vi "Forebrain - Final.vi"() -> ()   [LabVIEW 2012]
doc: "This VI contrains the Forebrain within the Olin Robot Architecture. It must be run first to load the appropriate mission definition files. It contains a finite state machine built around a tabbed Operator interface that will guide an operator through the startup, run shutdown mission sequence. After running it, run the Midbrain and Hindbrain VIS."
panel:
  in  "Batshit Velocity":i16
  in  "Alt Rudder":dbl=10.0
  in  "Default Rudder":dbl=9.0
  in  "Max Radius":dbl=300.0
  in  "Battshit":bool
  out "Battery Level":dbl
  in  "MapDarWithBuoys?":bool
  out "under cloud?":bool
  out "WhatAroundMeMap? Filtered":cluster{"T":dbl, "Range":dbl, "Bearing":dbl}[](array[cluster])
  out "Forebrain to Midbrain":T1
  in  "Upper Midbrain Active":bool=TRUE
  out "Ir distance":i16
  in  "Midbrain Behavior weights":i8[](array[numeric])=[10, 0, 0, 0, 0, 0]
  in  "SOFT E-STOP":bool
  in  "Upper Midbrain Tweaks":T2={"Lider good scale mult"=0.00125, "Lider good scale add"=0.0, "Lider speed scale mult"=0.018, "Lider speed scale add"=0.0, "Follow right?"=FALSE, "IR Following Distance"=400, "IR scaling div"=50.0, "Lidar Cutoff"=0.0}
  out "Normalized Buoy Array":i32[][](array[numeric])
  in  "Buoy Array":i32[][](array[numeric])
  out "Number Waypoints":i32
  out "NXT String Sent":string="$B^"
  in  "Soft E-Stop":bool
  out "NXT String Received":string
  out "return count":u32
  out "error out":errorcluster
  in  "error in 2":errorcluster
  out "Desired \nVelocity":i16=5
  out "Ycurrent":dbl format="%#_3g"
  out "Xcurrent":dbl format="%#_3g"
  out "Ystart":dbl
  out "Xstart":dbl
  in  "error in":errorcluster
  out "Robot Live":bool
  in  "E-Stop":bool
  in  "Tab":T3(tab)
  out "MissionTime (Min)":dbl(knob) scale=0.0..10.0
  out "LidarDist":i16
  out "IR Index":i32
  out "BatteryLevel":dbl(slide) scale=6.0..9.0
  out "String Received":string
  out "Send String":string="$B^"
  in  "VISA resource name":refnum<visa-resource-name>="COM6"
  in  "Mode":i16 min=0 max=99 step=1
  in  "Desired Vel":i16(slide)=7 scale=0.0..14.0
  in  "Local Head":i16(slide)=7 scale=0.0..14.0
  out "StartMissionMap":picture
  out "MapDARCheck":picture
  in  "RunRobot":bool
  in  "Tug letter":string="T"
  out "Tug X":i32
  out "Tug Y":i32
  out "Tug H":i32
  out "BS Time Out?":bool
  out "Buoy locations":cluster{"regular expression":string, i32, i32}[](array[cluster])
  out "Valid ?":bool
  out "Battery\nVolts":i16
  out "Base Station data rec'd":string
  out "udp rate":bool
  out "CollisionWarning":bool
  out "DebugMapDAR":picture
  in  "MapDAR Control":T4={"NumberOfBeams"=180, "SensorRange"=500.0, "Noise (0.1 to 1)"=0.0} {"Noise (0.1 to 1)" min=0.0 max=1.0 step=0.1; "SensorRange" min=500.0 max=1500.0 step=100.0; "NumberOfBeams" min=36 max=360 step=2}
  out "MapDAR Data (r:pixel b:degrees)":cluster{"Range":dbl, "Bearing":dbl}[](array[cluster])
  in  "Stop DebugSENSE":bool
  out "MissionMap":picture
  out "Tug position":T5
  out "initialized MDF":T6(array[cluster])
  out "Way Point Index":i32
  out "InitialWaypoint":cluster{"X":i16, "Y":i16}
  in  "Pen Color":u32(colorbox)=15671808
  in  "Select Pen Attributes":T7={"Width"=1, "Style"=enum."Solid"}
  out "Draw??":bool
  in  "WhereAmI?FromBase":T8
  out "(xr,yr)":cluster{"X":dbl, "Y":dbl}
  in  "RobotPosition":T5 {"xrobot" min=0.0 max=1177.0 step=10.0; "yrobot" min=0.0 max=850.0 step=10.0; "heading" min=0.0 max=7.0 step=0.1}
  out "MDF_Original":T6(array[cluster])
  out "WhatAroundMeMap?":cluster{"T":dbl, "Range":dbl, "Bearing":dbl}[](array[cluster])
  out "WayPointAct":dbl[](array[numeric])
  out "SteerAngle":dbl
  out "MissionDefFile":picture
  out "MDF":T6(array[cluster])
  in  "Select Your Behavior":T9(ring)
  out "No. of Waypoints":i32
  in  "Exit Planning":bool
  in  "BoatSpeed for Leg":dbl(slide)=8.0 min=-9.0 max=9.0 step=1.0 scale=0.0..14.0
  out "BuildMDF":bool
  out "WayPoint Position":cluster{"X":i32, "Y":i32}
  out "Send String to NXT":string="$B^"
  in  "Behavior Command":T9(ring)
  out "CollisionLight":bool
  out "Where? Manual":T8
  out "ActManual":bool
  in  "Manual Heading":i16(knob)=7 min=0 max=14 step=1
  out "MWhat?":bool
  out "Where? 2":bool
  out "How? 2":bool
  in  "ManualModeStop":bool
  out "ManualModeMapDAR":picture
  out "ManualMissionMap":picture
  out "Battery":dbl(slide) scale=0.0..8.0
  in  "Manual Vel":dbl(slide)=7.0 min=0.0 max=14.0 step=1.0 scale=0.0..14.0
  out "MissionTime":dbl(knob) scale=0.0..10.0
  out "Heading":cluster{dbl, dbl}(knob)={0.0, 34.390870865624734} scale=180.0..-179.0 scale format="%#_3g"
  out "Speed":i16(knob) scale=-6.0..6.0
  out "Current Behavior":T9(ring)
  out "Robot Position":cluster{"X":dbl, "Y":dbl} {"X" format="%#_3g"; "Y" format="%#_3g"}
  out "Ready":bool
  in  "Pause":bool
  in  "Rerun MDF":bool
  out "CollisionLight 2":bool
  out "Act":bool
  out "Neo-C":bool
  out "How?":bool
  out "What?":bool
  out "A Heading":cluster{dbl, dbl}(knob)={0.0, 34.390870865624734} scale=180.0..-180.0
  out "A Speed":dbl(knob) scale=-9.0..9.0
  out "AutoBattery":dbl(slide) scale=0.0..8.0
  out "AutoModeLIDAR":picture
  out "AutoMissionMap":picture
  in  "RunAutoMode":bool
  out "MissionTimeAuto":dbl(knob) scale=0.0..60.0
  out "Where?":bool
  in  "MISSION NUMBER (1 OR 2)":dbl=1.0
  in  "Mission 2":i64[][](array[numeric])=[[0, 525, 450, 525], [50, 275, 250, 275], [240, 250, 650, 250], [500, 605, 900, 650], [550, 940, 700, 940]]
  in  "WAYPOINT MODE":dbl=1.0
  in  "Current Waypoint":dbl
  in  "Manual\nOverride":bool=TRUE
  in  "Mission 1":i64[][](array[numeric])=[[120, 280, 700, 408], [30, 280, 250, 400], [100, 575, 450, 575], [175, 950, 600, 950]]
  out "BAM Mission Map":picture
  out "Pixel X":dbl
  out "Pixel Y":dbl
  out "Direction":dbl
  out "Base Station String":string
  in  "Heading":i16(knob)=7
  in  "Velocity":i16(slide)=7 scale=0.0..14.0
  out "Local\nHeading":i16=90
  # "To run\nrobot,\nclick\narrow\nabove\n\nRun Robot button must be on"
  # "Operation Directions\n\n1)Click on Startup&\nShutdown tab.\n2) Click on Run \nArrow on menubar.\nRun Forebrain,\nvis from the project\nexplorer.\n3) Select a mssion \nmap file when asked.\n4) Check robot is \nfully operational on\nStartup tab.\n5) Debug with debug\ntabs as required.\n6) Select ManualMode\ntab and test drive \nrobot.\n7) Select PlanMission\ntab and set up \nmission.\n8) Go to AutoMode\ntab and run mission."
  # "BATSHIT PROTOCOL"
  # "Turns off drive\nmotors"
  # "forebrain"
  # "wall follow"
  # "wall avoid"
  # "under cloud"
  # "GTFO"
  # "tend straight"
  # "IR wall avoid"
  # "inactive behaviors = 0\nstrongest behavior = 10"
  # "under cloud should always be zero"
  # "under cloud?"
  # "Enter Olin Test  Pool"
  # "Xbee Com Port"
  # "xBee\"Send String\" (mode, desired velocity, local heading)"
  # "(Type in Tug Letter  L T G P  (look at boat cradle)"
  # "Should be on to\nrun"
  # "BoatG,X,Y,H,BoatT,X,Y,H,BoatP,X,Y.H,BoatL,X,Y,H,BuoyA,X,Y,BuoyB,X,Y,BuoyC,X,Y,BuoyD,X,Y,Time(hours,Min,Sec)"
  # "To stop  program \nturn off here"
  # "Use this tab\nto explore\nLIDAR\ndata and \noperation"
  # "Set\nNumberOfBeams\nSensorRange\nNoise\nto\nview\nsimulated\nsensor\ndata"
  # "Turn Debug Sim \nto leave this\ntab--->"
  # "This tab will auto\nreturn to Startup \nin 2 seconds"
  # "Clean up interface and make more useful for debugging behaviors"
  # "Build out interface and make more useful for debugging act"
  # "This tab will auto\nreturn to Startup \nin 2 seconds"
  # "Directions:\n1) Select Robot Behavior for each mission leg.\n2) Select Robot Speed for leg.\n3) Click on robots current location for first waypoint.\n4) Hold down button and drag to next\nwaypoint. Click on next leg waypoint.\n5) Hold mouse button down and drag to \nnext waypoint. \n6) Click on next waypoint. Repeat for full mission.\n7) MDF will store up to 20 waypoints."
  # "Remember to\nset boat\nleg speed !"
  # "Please Adjust Scroll Barrs in Tug Off Mode to Prevent  Extra Lines Being Drawn"
  # "\"Send String\" (mode, desired velocity, local heading)"
  # "Press to stop and return to StartUp"
  # "Open MidBrain\nArbiter to see\nBrain Waves"
  # "AutoMode\nAutomatically \nReturns to \nStartUp Mode"
  # "LOCATION"
  # "MANUAL CONTROL"
  # "Pixel coordinates for destinations."
  # "BoatG,X,Y,H,BoatT,X,Y,H,BoatP,X,Y.H,BoatL,X,Y,H,BuoyA,X,Y,BuoyB,X,Y,BuoyC,X,Y,BuoyD,X,Y,Time(hours,Min,Sec)"
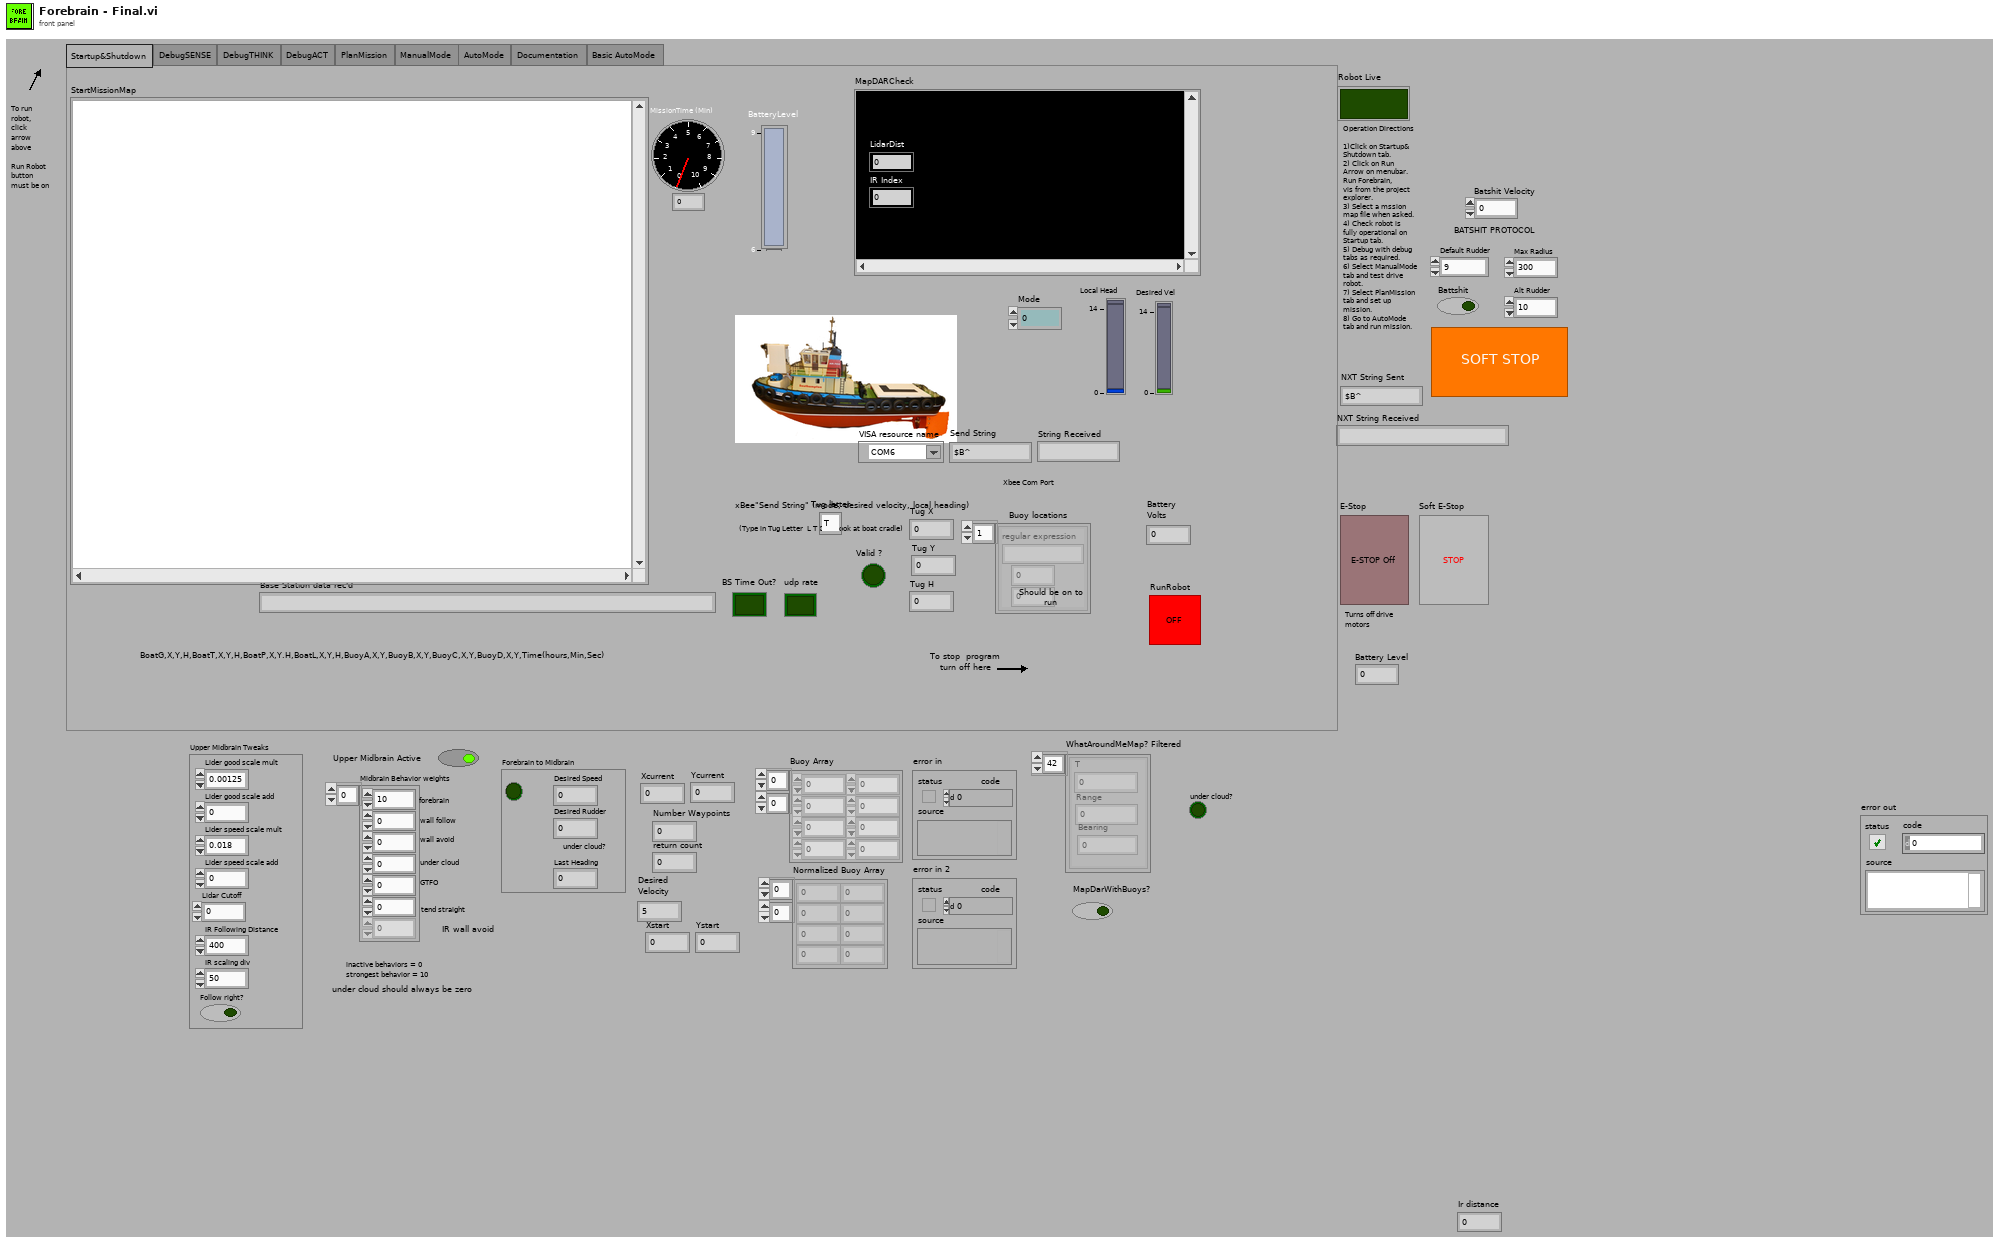
[diagram p1: front panel]
types:
  T1 = cluster{"Desired Speed":i16, "Desired Rudder":i16, bool, "Last Heading":i16}
  T2 = cluster{"Lider good scale mult":dbl, "Lider good scale add":dbl, "Lider speed scale mult":dbl, "Lider speed scale add":dbl, "Follow right?":bool, "IR Following Distance":i32, "IR scaling div":dbl, "Lidar Cutoff":dbl}
  T3 = enum32{"Startup&Shutdown", "DebugSENSE", "DebugTHINK", "DebugACT", "PlanMission", "ManualMode", "AutoMode", "Documentation", "Basic AutoMode"}
  T4 = cluster{"NumberOfBeams":i32, "SensorRange":dbl, "Noise (0.1 to 1)":dbl}
  T5 = cluster{"xrobot":dbl, "yrobot":dbl, "heading":dbl}
  T6 = cluster{"Status":enum16{"Past", "Current", "Future"}, "x":dbl, "y":dbl, "z":dbl, "Vel":dbl, "Dwell Time":dbl, "BehCom":enum16{"Tug Off", "Manual Mode", "Goto WayPoint", "Back Up", "Circle", "Left Wall Follow", "Right Wall Follow", "Hunt"}, "Expand1":dbl, "Expand2":dbl, "Expand3":dbl}[]
  T7 = cluster{"Width":u16, "Style":enum32{"Solid", "Dash", "Dot", "DashDot", "DashDotDot"}}
  T8 = cluster{"T":dbl, "X":dbl, "Y":dbl, "Direction":dbl}
  T9 = enum16{"Tug Off", "Manual Mode", "Goto WayPoint", "Back Up", "Circle", "Left Wall Follow", "Right Wall Follow", "Hunt"}
  T10 = enum32{"Startup&Shutdown", "DebugSENSE", "DebugTHINK", "DebugACT", "PlanMission", "ManualMode", "AutoMode", "Documentation"}
  T11 = cluster{"VelCom":dbl, "BehCom":enum16{"OpenFieldTransit", "P-WallFollow", "S-WallFollow", "LaneFollow", "ManualMode"}}
  T12 = typedef "IMAQ Image.ctl" = refnum<image>
  T13 = typedef "imagedata.ctl" = cluster{"image type":i32, "image depth":i32, "image":u8[], "mask":u8[], "colors":u32[], "Rectangle":cluster{"left":i16, "top":i16, "right":i16, "bottom":i16}}
  T14 = cluster{"Status":enum16{"Past", "Current", "Future"}, "x":dbl, "y":dbl, "z":dbl, "Vel":dbl, "Dwell Time":dbl, "BehCom":enum16{"Tug Off", "Manual Mode", "Goto WayPoint", "Back Up", "Circle", "Left Wall Follow", "Right Wall Follow", "Hunt"}, "Expand1":dbl, "Expand2":dbl, "Expand3":dbl}
  T15 = typedef "LVMouseTypeDef.ctl" = cluster{"Mouse Position":cluster{"X":i32, "Y":i32}, "Mouse Modifiers":cluster{"Button Down":bool, "Shift Mod":bool, "Menu Mod":bool, "Option Mod":bool}}
  T16 = cluster{"RudderAngle":i16, "t":i16, "under cloud?":bool, "RudderAngle":i16}
  T17 = cluster{"regular expression":string, i32, i32, i32}
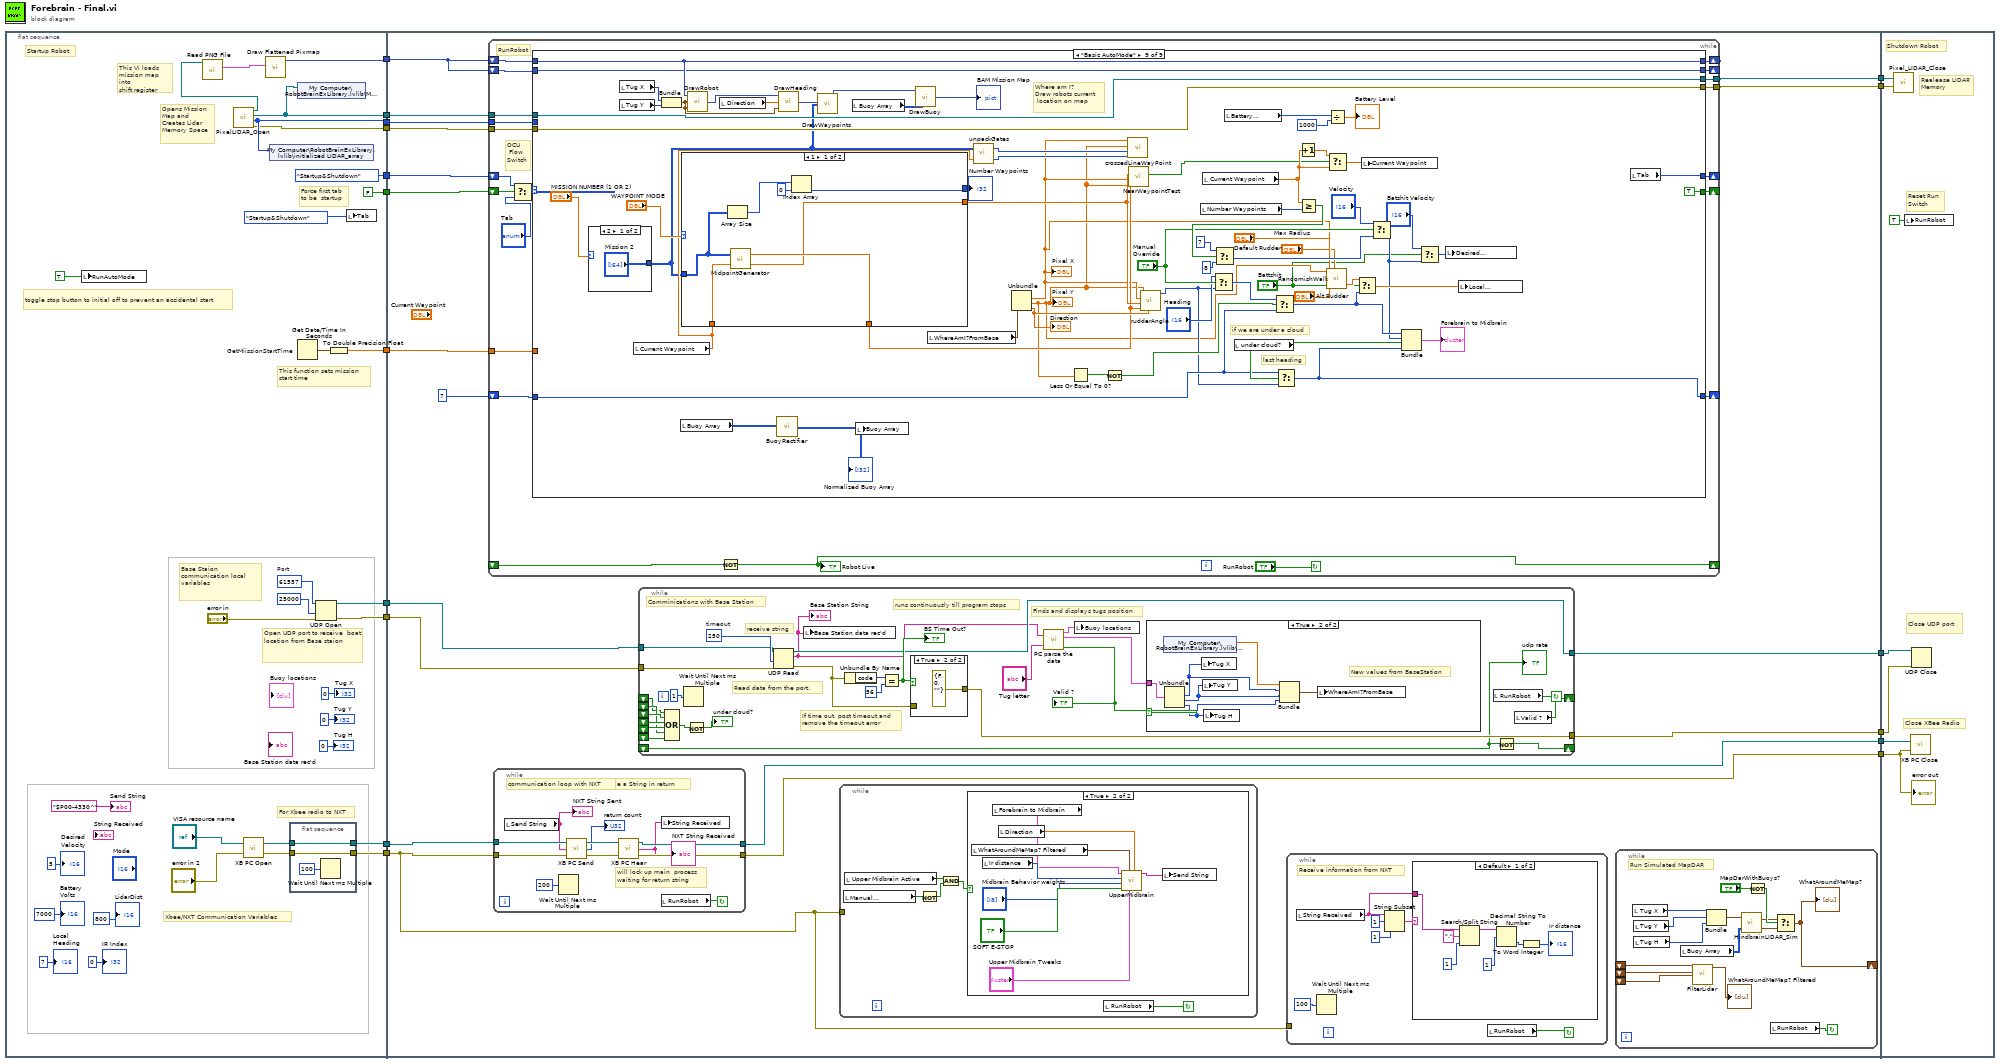
[diagram p0: block diagram]
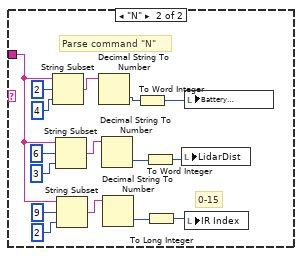
[diagram p2: hidden frame]
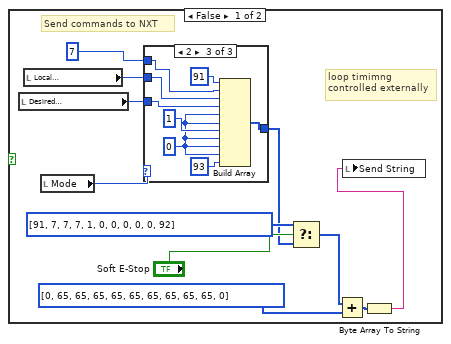
[diagram p3: hidden frame]
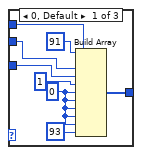
[diagram p4: hidden frame]
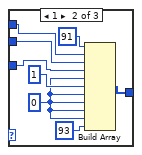
[diagram p5: hidden frame]
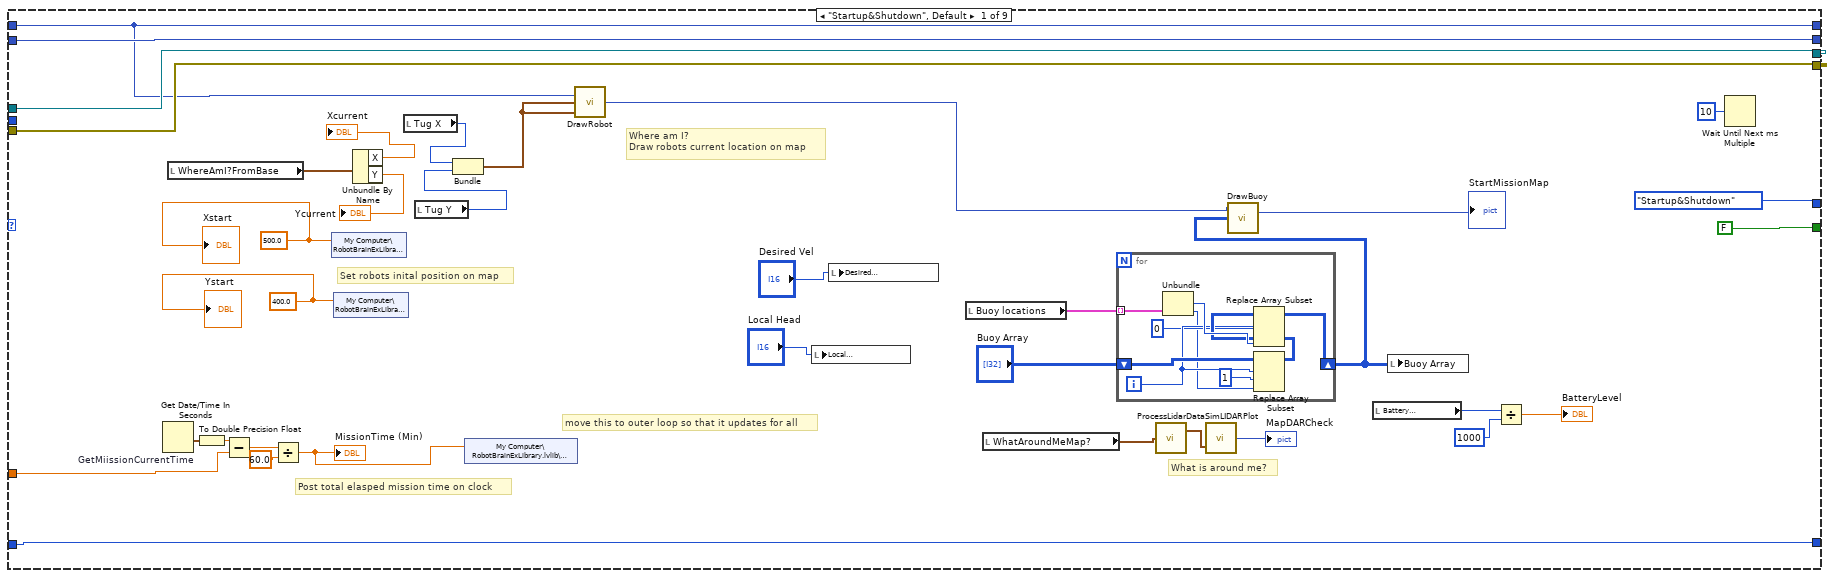
[diagram p8: hidden frame]
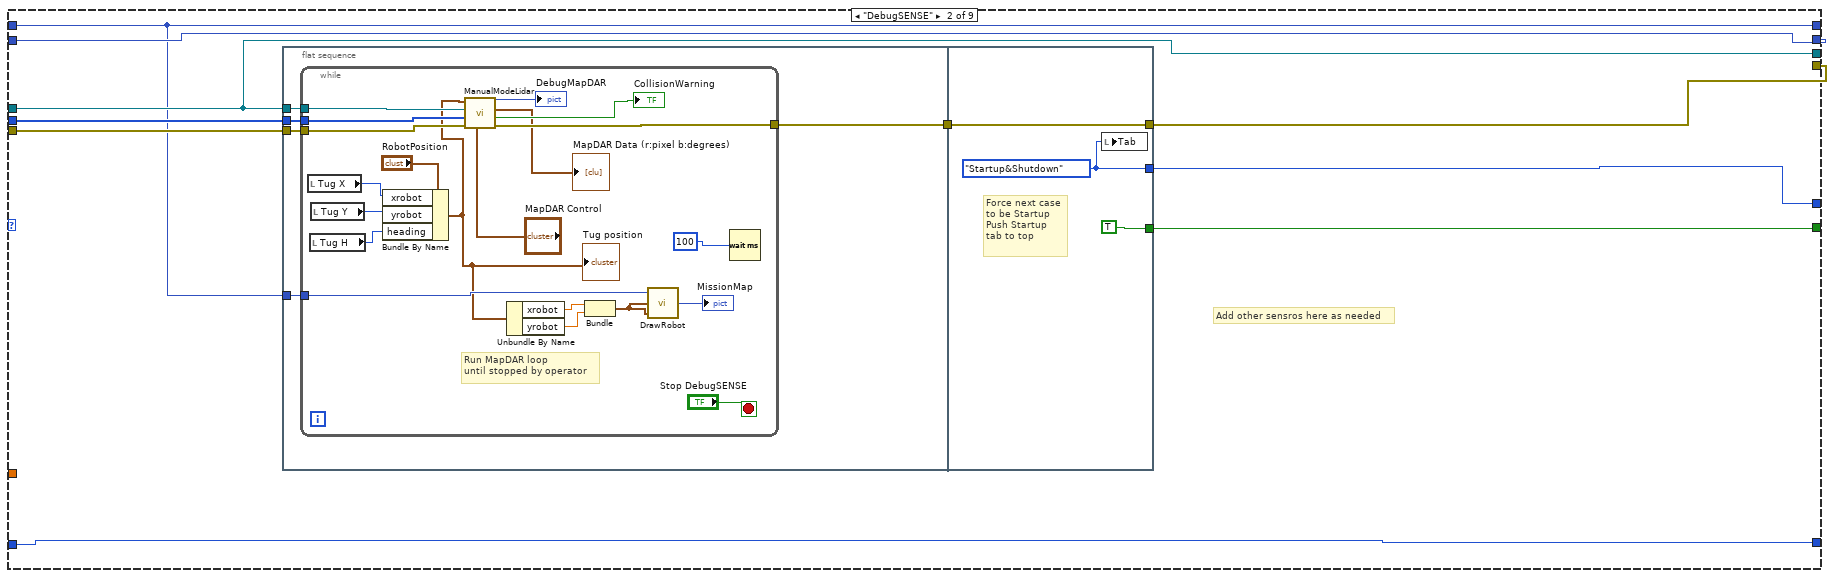
[diagram p9: hidden frame]
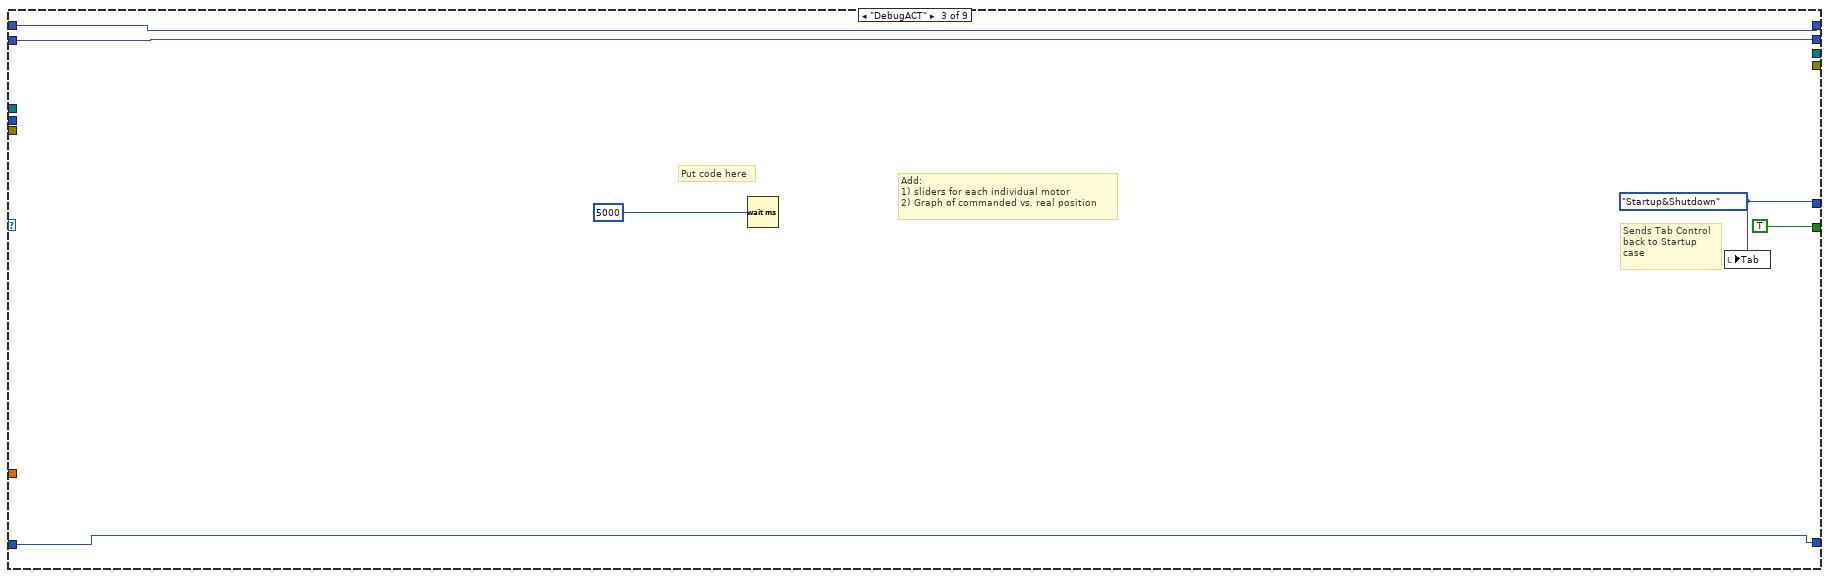
[diagram p10: hidden frame]
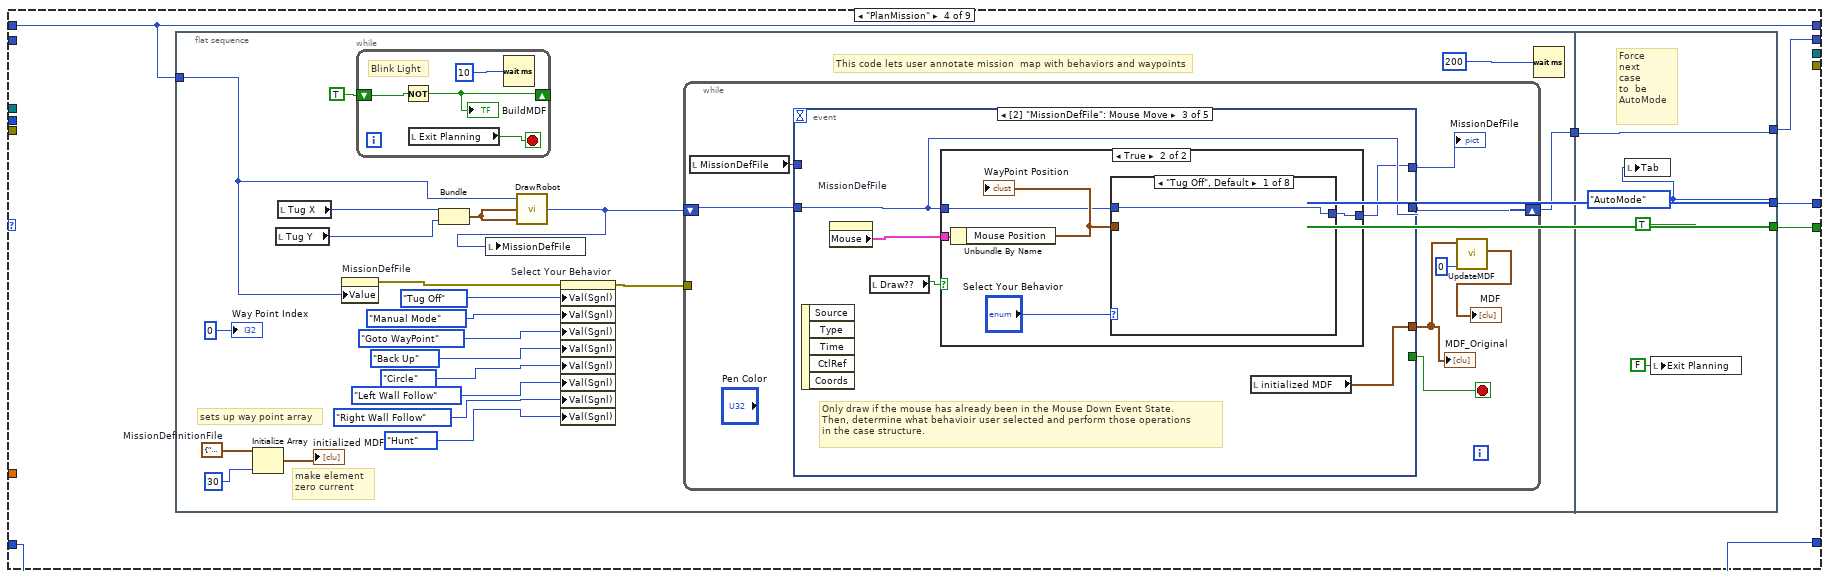
[diagram p11: hidden frame]
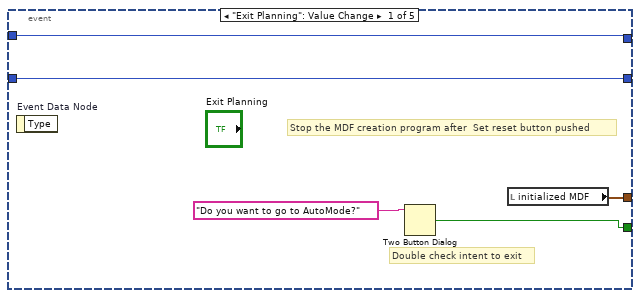
[diagram p12: hidden frame]
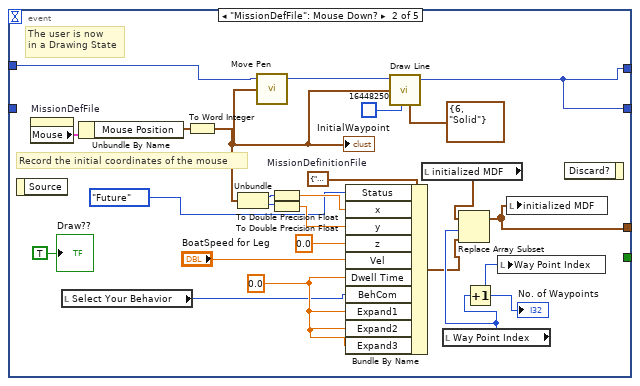
[diagram p13: hidden frame]
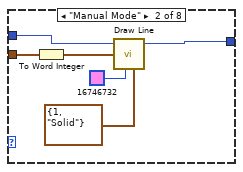
[diagram p15: hidden frame]
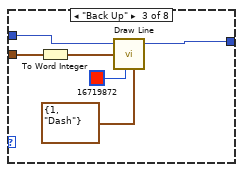
[diagram p16: hidden frame]
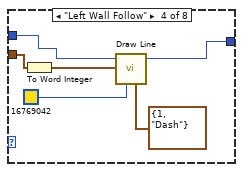
[diagram p17: hidden frame]
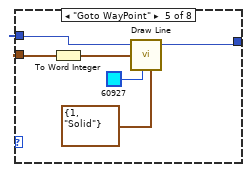
[diagram p18: hidden frame]
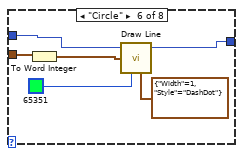
[diagram p19: hidden frame]
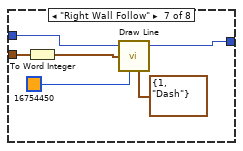
[diagram p20: hidden frame]
diagram:
  n1 = flat-sequence {
    tunnel: [w48] -> w17
    tunnel: [w47] -> w16
    tunnel: [w44] -> w15
    tunnel: [w46] -> w14
    tunnel: [w45] -> w13
    tunnel: [FALSE ("RunAutoMode")] -> w10
    tunnel: [T10."Startup&Shutdown" ("Tab")] -> w9
    tunnel: [w31] -> w8
    tunnel: [w30] -> w7
    tunnel: [w19] -> w6
    tunnel: [w18] -> w5
    tunnel: w17 -> [w70]
    tunnel: w16 -> [w69]
    tunnel: w15 -> [w68]
    tunnel: w14 -> [w67]
    tunnel: w13 -> [w66]
    tunnel: [w65] -> w12
    tunnel: [w64] -> w11
    tunnel: w10 -> [w63]
    tunnel: w9 -> [w62]
    tunnel: w8 -> [w57]
    tunnel: w7 -> [w56]
    tunnel: w6 -> [w61]
    tunnel: w5 -> [w58]
    tunnel: [w60] -> w4
    tunnel: [w59] -> w3
    tunnel: [w55] -> w2
    tunnel: [w54] -> w1
    tunnel: w12 -> [w756]
    tunnel: w11 -> [w755]
    tunnel: w4 -> [w754]
    tunnel: w3 -> [w753]
    tunnel: w2 -> [w752]
    tunnel: w1 -> [w751]
    frame #0 {
      w37 = u16 61557  # Port
      # "For Xbee radio to NXT"
      # "Xbee/NXT Communication Variables"
      # "Base Staion communication local variables"
      # "Open UDP port to receive  boat location from Base staion"
      # "Force first tab\nto be  startup"
      # "toggle stop button to initial off to prevent an accidental start"
      # "Opens Mission\nMap and\nCreates Lidar\nMemory Space"
      # "This function sets mission \nstart time"
      # "This Vi loads\nmission map into \nshift register"
      # "Startup Robot"
      n2 = local write "RunAutoMode"(TRUE ("RunAutoMode")) -> ()
      n3 = call "PixelLIDAR_Open.vi"() -> ("error out"=w45:errorcluster, "initialized LIDAR\narray"=w46:i32[], "MDF Image"=w44:T12, "MissionMap"=w39:path)  [unwired: 2 in]
      n4 = call <vilib>:"Read PNG File.vi"("path to PNG file"=w39) -> ("image data"=w38:T13)  [unwired: 8 in, 2 out]
      n5 = call "XB PC Open.vi"("error in (no error)"="error in 2", "VISA resource name"="VISA resource name") -> ("error out"=w22:errorcluster, "VISA resource name out"=w23:refnum<visa-resource-name>)
      n6 = call <vilib>:"Draw Flattened Pixmap.vi"("image data"=w38) -> ("new picture"=w47:picture)  [unwired: 8 in]
      n7 = shared-variable "My Computer\\RobotBrainExLibrary.lvlib\\initialized LIDAR_array"(w46) -> ()  [unwired: 1 in, 1 out]
      n8 = flat-sequence {
        tunnel: w23 -> [w50]
        tunnel: w22 -> [w51]
        tunnel: [w51] -> w18
        tunnel: [w50] -> w19
        frame #0 {
          n9 = Wait Until Next ms Multiple(millisecond multiple=u32 100) -> ()  [unwired: 1 out]
        }
      }
      n10 = shared-variable "My Computer\\RobotBrainExLibrary.lvlib\\MDF Image"(w44) -> ()  [unwired: 1 in, 1 out]
      n11 = Get Date/Time In Seconds "GetMiissionStartTime"() -> (seconds since 1Jan1904=w49:timestamp)
      n12 = UDP Open(8:"error in", 9:25000 ("timeout ms (25000)"), 11:w37) -> (port=w31:refnum<k16>, 0:w30:errorcluster)  [unwired: 2 in, 1 out]
      n13 = To Double Precision Float(number=w49) -> (double precision float=w48:dbl)
      n14 = local write "Tab"(T10."Startup&Shutdown" ("Tab")) -> ()
      "Tug X" <- 0 ("Tug X")
      "Tug Y" <- 0 ("Tug Y")
      "Tug H" <- 0 ("Tug H")
      "Battery\nVolts" <- i16 7000 ("Battery\nVolts")
      "LidarDist" <- i16 800 ("Dist")
      "IR Index" <- 0 ("IR Index")
      "Local\nHeading" <- i16 7 ("Local\nHeading")
      "Desired \nVelocity" <- i16 5 ("Desired \nVelocity")
      "Send String" <- "$P00-4330^"
    }
    frame #1 {
      n15 = while {
        shift-right: [w212] -> _
        shift-left: _ -> [w228]
        shift-right: [w227] -> _
        shift-left: w62 -> [w226]
        shift-right: [w223] -> _
        shift-left: w63 -> [w222]
        tunnel: w70 -> [w221]
        shift-right: [w211] -> _
        shift-left: w69 -> [w220]
        shift-right: [w218] -> _
        shift-left: w69 -> [w219]
        tunnel: w68 -> [w217]
        tunnel: w67 -> [w216]
        tunnel: w66 -> [w215]
        tunnel: [w214] -> w65
        tunnel: [w213] -> w64
        shift-right: [w210] -> _
        shift-left: i16 7 ("Heading") -> [w209]
        stop <- "RunRobot" continue-if-true
        # "RunRobot"
        # "OCU\n Flow\nSwitch"
        n16 = Select(t=w226, s=w222, f="Tab") -> (s? t:f=w224:T3)
        n17 = case shown="\"Basic AutoMode\"" w224 {
          selector: w224 -> [_ _ _ _ _ w567 _ _ _]
          tunnel: [T10."Startup&Shutdown" ("Tab") w279 w315 w323 w491 w568 T10."Startup&Shutdown" ("Tab") w666 w720] -> w227
          tunnel: [FALSE ("s") w278 TRUE ("s") w322 w492 w566 FALSE ("s") TRUE ("s") TRUE ("s")] -> w223
          tunnel: w221 -> [w258 _ _ _ w489 w564 _ _ _]
          tunnel: w220 -> [w236 w275 w314 w319 w487 w561 w658 w664 w726]
          tunnel: w219 -> [w257 w276 w313 _ w488 w563 w657 w663 w725]
          tunnel: [w257 w276 w313 w320 w488 w563 w657 w663 w725] -> w218
          tunnel: w217 -> [w256 w277 _ _ _ _ _ _ w721]
          tunnel: w216 -> [_ w283 _ _ _ _ _ _ _]
          tunnel: w215 -> [w255 w282 _ _ _ _ _ _ w718]
          tunnel: [w256 w277 _ _ _ _ _ _ w721] -> w214
          tunnel: [w255 w281 _ _ _ _ _ _ w718] -> w213
          tunnel: [w236 w275 w314 w319 w487 w561 w658 w664 w726] -> w211
          tunnel: [w230 w274 w312 w318 w486 w560 w656 w662 w694] -> w210
          tunnel: w209 -> [w230 w274 w312 w318 w486 w560 w656 w662 w685]
          frame "Startup&Shutdown", Default {
            w247 = 400.0 ("Ystart")
            w248 = 500.0 ("Xstart")
            # "move this to outer loop so that it updates for all"
            # "Where am I?\nDraw robots current location on map"
            # "Post total elasped mission time on clock"
            # "What is around me?"
            # "Set robots inital position on map"
            n18 = Get Date/Time In Seconds "GetMiissionCurrentTime"() -> (seconds since 1Jan1904=w262:timestamp)
            n19 = local read "WhereAmI?FromBase"() -> (w237:T8)
            n20 = To Double Precision Float(number=w262) -> (double precision float=w261:dbl)
            n21 = Subtract(x=w261, y=w258) -> (x-y=w260:dbl)
            n22 = Divide(x=w260, y=60.0) -> (x/y=w254:dbl)
            "MissionTime (Min)" <- w254
            n23 = shared-variable "My Computer\\RobotBrainExLibrary.lvlib\\Xstart"(w248) -> ()  [unwired: 1 in, 1 out]
            n24 = shared-variable "My Computer\\RobotBrainExLibrary.lvlib\\Ystart"(w247) -> ()  [unwired: 1 in, 1 out]
            n25 = Unbundle By Name(w237) -> ("X"=→"Xcurrent":dbl, "Y"=→"Ycurrent":dbl)
            n26 = local read "Tug X"() -> (w246:i32)
            n27 = local read "Tug Y"() -> (w245:i32)
            n28 = Bundle("Tug X"=w246, "Tug Y"=w245) -> (w251:cluster{"Tug X":i32, "Tug Y":i32})  [unwired: 1 in]
            n29 = shared-variable "My Computer\\RobotBrainExLibrary.lvlib\\MissionTime"(w254) -> ()  [unwired: 1 in, 1 out]
            n30 = call "DrawRobot.vi"("(xr,yr) old"=w251, "(xr,yr) new"=w251, "2D Picture"=w236) -> ("new picture"=w235:picture)
            n31 = local write "Local\nHeading"("Local Head") -> ()
            n32 = local write "Desired \nVelocity"("Desired Vel") -> ()
            n33 = local read "Buoy locations"() -> (w233:cluster{"regular expression":string, i32, i32}[])
            n34 = local read "WhatAroundMeMap?"() -> (w238:cluster{"T":dbl, "Range":dbl, "Bearing":dbl}[])
            n35 = for {
              tunnel: w233 -> [w273] mode=indexing
              shift-right: [w269] -> w231
              shift-left: "Buoy Array" -> [w272]
              i -> [w267]
              n36 = Unbundle(w273) -> (w271:i32, w265:i32)  [unwired: 1 out]
              n37 = Replace Array Subset(array=w272, new element=w265, index (row)=w267, index (col)=1 ("index")) -> (w270:i32[][])
              n38 = Replace Array Subset(array=w270, new element=w271, index (row)=w267, index (col)=0 ("index")) -> (w269:i32[][])
            }
            n39 = call "ProcessLidarData.vi"("WhatAroundMe?MM"=w238) -> ("data array [mag, phase (deg)]"=w252:cluster{"magnitude":dbl, "phase":dbl}[])  [unwired: 1 out]
            n40 = call "SimLIDARPlot.vi"("data array [mag, phase (deg)]"=w252) -> ("SONAR"=→"MapDARCheck":picture)  [unwired: 1 in]
            n41 = call "DrawBuoy.vi"("Array"=w231, "2D Picture"=w235) -> ("new picture"=→"StartMissionMap":picture)  [unwired: 1 in]
            n42 = local read "Battery\nVolts"() -> (w242:i16)
            n43 = local write "Buoy Array"(w231) -> ()
            n44 = Divide(x=w242, y=i16 1000) -> (x/y=→"BatteryLevel":dbl)
            n45 = Wait Until Next ms Multiple(millisecond multiple=u32 10) -> ()  [unwired: 1 out]
            "Xstart" <- w248
            "Ystart" <- w247
          }
          frame "DebugSENSE" {
            # "Add other sensros here as needed"
            n46 = flat-sequence {
              tunnel: w283 -> [w288]
              tunnel: w282 -> [w287]
              tunnel: w277 -> [w286]
              tunnel: [w285] -> w280
              tunnel: w275 -> [w284]
              tunnel: [w311] -> w281
              tunnel: w280 -> [w311]
              tunnel: [w310] -> w279
              tunnel: [TRUE ("s")] -> w278
              frame #0 {
                n47 = while {
                  tunnel: w288 -> [w308]
                  tunnel: w287 -> [w307]
                  tunnel: w286 -> [w306]
                  tunnel: [w305] -> w285
                  tunnel: w284 -> [w299]
                  stop <- "Stop DebugSENSE" stop-if-true
                  # "Run MapDAR loop\nuntil stopped by operator"
                  n48 = local read "Tug X"() -> (w293:i32)
                  n49 = local read "Tug H"() -> (w294:i32)
                  n50 = local read "Tug Y"() -> (w292:i32)
                  n51 = Bundle By Name(cluster="RobotPosition", "xrobot"=w293, "yrobot"=w292, "heading"=w294) -> (w290:T5)
                  "Tug position" <- w290
                  n52 = call "ManualModeLidar.vi"("LIDARControl"="MapDAR Control", "error in"=w307, "initialized \nsonar ray\narray"=w308, "MDF Image"=w306, "SubPosition"=w290) -> ("error out"=w305:errorcluster, "Collision\nWarning"=→"CollisionWarning":bool, "LIDAR Data (r:pixel b:degrees)"=→"MapDAR Data (r:pixel b:degrees)":cluster{"Range":dbl, "Bearing":dbl}[], "LIDAR"=→"DebugMapDAR":picture)  [unwired: 1 in]
                  n53 = Unbundle By Name(w290) -> ("xrobot"=w297:dbl, "yrobot"=w296:dbl)
                  n54 = Bundle("xrobot"=w297, "yrobot"=w296) -> (w289:cluster{"xrobot":dbl, "yrobot":dbl})  [unwired: 1 in]
                  n55 = call "DrawRobot.vi"("(xr,yr) old"=w289, "(xr,yr) new"=w289, "2D Picture"=w299) -> ("new picture"=→"MissionMap":picture)
                  n56 = Wait (ms)(milliseconds to wait=u32 100) -> ()  [unwired: 1 out]
                }
              }
              frame #1 {
                w310 = T10."Startup&Shutdown" ("Tab")
                # "Force next case\nto be Startup\nPush Startup\ntab to top"
                n57 = local write "Tab"(w310) -> ()
              }
            }
          }
          frame "DebugACT" {
            w315 = T10."Startup&Shutdown" ("Tab")
            # "Add:\n1) sliders for each individual motor\n2) Graph of commanded vs. real position"
            # "Put code here"
            # "Sends Tab Control\nback to Startup\ncase"
            n58 = Wait (ms)(milliseconds to wait=u32 5000) -> ()  [unwired: 1 out]
            n59 = local write "Tab"(w315) -> ()
          }
          frame "PlanMission" {
            n60 = flat-sequence {
              tunnel: [w344] -> w321
              tunnel: w319 -> [w337]
              tunnel: [w484] -> w323
              tunnel: [TRUE ("s")] -> w322
              tunnel: w321 -> [w483]
              tunnel: [w483] -> w320
              frame #0 {
                w335 = T14 {"Status"=enum."Future", "x"=0.0, "y"=0.0, "z"=0.0, "Vel"=0.0, "Dwell Time"=0.0, "BehCom"=enum."Tug Off", "Expand1"=0.0, "Expand2"=0.0, "Expand3"=0.0}  # MissionDefinitionFile
                # "make element \nzero current"
                # "sets up way point array"
                # "This code lets user annotate mission  map with behaviors and waypoints"
                n61 = Initialize Array ("Initialize WaypointArray")(w335, 30 ("dimension size")) -> (→"initialized MDF":T6)
                n62 = local read "Tug Y"() -> (w332:i32)
                n63 = local read "Tug X"() -> (w333:i32)
                n64 = property on="MissionDefFile" class="Pict"("Value"=w337) -> (error out=w342:errorcluster)  [unwired: 2 in, 1 out]
                n65 = while {
                  shift-right: [w348] -> _
                  shift-left: TRUE -> [w349]
                  stop <- w347 stop-if-true
                  # "Blink Light"
                  n66 = Not(x=w349) -> (.not. x?=w348:bool)
                  "BuildMDF" <- w348
                  n67 = local read "Exit Planning"() -> (w347:bool)
                  n68 = Wait (ms)(milliseconds to wait=u32 10) -> ()  [unwired: 1 out]
                }
                n69 = Bundle("Tug X"=w333, "Tug Y"=w332) -> (w338:cluster{"Tug X":i32, "Tug Y":i32})  [unwired: 1 in]
                n70 = call "DrawRobot.vi"("(xr,yr) old"=w338, "(xr,yr) new"=w338, "2D Picture"=w337) -> ("new picture"=w336:picture)
                n71 = local write "MissionDefFile"(w336) -> ()
                n72 = property on="Select Your Behavior" class="Enum (strict)"(error in=w342, "Val(Sgnl)"=T9."Tug Off" ("Value (Signaling)"), "Val(Sgnl)"=T9."Manual Mode" ("Value (Signaling)"), "Val(Sgnl)"=T9."Goto WayPoint" ("Value (Signaling)"), "Val(Sgnl)"=T9."Back Up" ("Value (Signaling)"), "Val(Sgnl)"=T9."Circle" ("Value (Signaling)"), "Val(Sgnl)"=T9."Left Wall Follow" ("Value (Signaling)"), "Val(Sgnl)"=T9."Right Wall Follow" ("Value (Signaling)"), "Val(Sgnl)"=T9."Hunt" ("Value (Signaling)")) -> (error out=w343:errorcluster)  [unwired: 1 in, 1 out]
                n73 = while {
                  shift-right: [w356] -> w344
                  shift-left: w336 -> [w357]
                  tunnel: w343 -> [_]
                  stop <- w355 stop-if-true
                  n74 = local read "MissionDefFile"() -> (w354:picture)
                  n75 = event shown="[2] \"MissionDefFile\": Mouse Move" {
                    selector: _ -> [_ _ _ _ _]
                    dyn-events: _ -> [_ _ _ _ _]
                    timeout: _ -> [_ _ _ _ _]
                    tunnel: [w360 w368 w388 w441 w479] -> w356
                    tunnel: w357 -> [w360 _ w388 w441 _]
                    tunnel: [w361 _ _ _ _] -> w355
                    tunnel: [w359 w383 w389 w443 w480] -> w351
                    tunnel: w354 -> [w358 w369 _ w442 w479]
                    tunnel: [w358 w368 w387 w442 w479] -> w353
                    event "Exit Planning": Value Change {
                      # "Double check intent to exit"
                      # "Stop the MDF creation program after  Set reset button pushed"
                      n76 = event-data "Event Data Node"() -> ()  [unwired: 1 in, 1 out]
                      n77 = Two Button Dialog(message="Do you want to go to AutoMode?") -> (T button?=w361:bool)  [unwired: 2 in]
                      n78 = local read "initialized MDF"() -> (w359:T6)
                    }
                    event "MissionDefFile": Mouse Down? {
                      w367 = T14 {"Status"=enum."Future", "x"=0.0, "y"=0.0, "z"=0.0, "Vel"=0.0, "Dwell Time"=0.0, "BehCom"=enum."Tug Off", "Expand1"=0.0, "Expand2"=0.0, "Expand3"=0.0}  # MissionDefinitionFile
                      w377 = 0.0 ("Dwell Time")
                      # "Record the initial coordinates of the mouse"
                      # "The user is now\nin a Drawing State"
                      n79 = event-data() -> ()  [unwired: 1 in, 1 out]
                      n80 = property on="MissionDefFile" class="Pict"() -> ("Mouse"=w386:T15)  [unwired: 2 in, 2 out]
                      n81 = local read "Select Your Behavior"() -> (w364:T9)
                      n82 = Unbundle By Name(w386) -> ("Mouse Position"=w384:cluster{"X":i32, "Y":i32})
                      n83 = To Word Integer(number=w384) -> (16bit integer=w372:cluster{"X":i16, "Y":i16})
                      "InitialWaypoint" <- w372
                      n84 = Unbundle(w372) -> ("X"=w381:i16, "Y"=w380:i16)
                      n85 = call <vilib>:"Move Pen.vi"("new position"=w372, "picture"=w369) -> ("new picture"=w373:picture)  [unwired: 3 in]
                      n86 = To Double Precision Float(number=w381) -> (double precision float=w379:dbl)
                      n87 = To Double Precision Float(number=w380) -> (double precision float=w378:dbl)
                      n88 = Bundle By Name(cluster=w367, "Status"=enum16{"Past", "Current", "Future"}."Future", "x"=w379, "y"=w378, "z"=0.0, "Vel"="BoatSpeed for Leg", "Dwell Time"=w377, "BehCom"=w364, "Expand1"=w377, "Expand2"=w377, "Expand3"=w377) -> (w363:T14)
                      n89 = call <vilib>:"Draw Line.vi"("picture"=w373, "end point"=w372, "color(black)"=u32 16448250, "pen"=T7 {"Width"=6, "Style"=enum."Solid"}) -> ("new picture"=w368:picture)  [unwired: 5 in]
                      n90 = local read "initialized MDF"() -> (w382:T6)
                      n91 = local read "Way Point Index"() -> (w365:i32)
                      n92 = Replace Array Subset(array=w382, new element=w363, index=w365) -> (w383:T6)
                      n93 = Increment(x=w365) -> (x+1=w385:i32)
                      "No. of Waypoints" <- w385
                      n94 = local write "Way Point Index"(w385) -> ()
                      n95 = local write "initialized MDF"(w383) -> ()
                      n96 = event-data() -> ()  [unwired: 2 in, 1 out]
                      "Draw??" <- TRUE ("Draw??")
                    }
                    event "MissionDefFile": Mouse Move {
                      # "Only draw if the mouse has already been in the Mouse Down Event State.\nThen, determine what behavioir user selected and perform those operations\nin the case structure."
                      n97 = event-data() -> ()  [unwired: 1 in, 5 out]
                      n98 = property on="MissionDefFile" class="Pict"() -> ("Mouse"=w391:T15)  [unwired: 2 in, 2 out]
                      n99 = local read "Draw??"() -> (w390:bool)
                      n100 = case shown="True" w390 {
                        tunnel: w391 -> [_ w397]
                        tunnel: w388 -> [w392 w393]
                        tunnel: [w392 w394] -> w387
                        frame False {
                        }
                        frame True {
                          n101 = Unbundle By Name(w397) -> ("Mouse Position"=w395:cluster{"X":i32, "Y":i32})
                          "WayPoint Position" <- w395
                          n102 = case shown="\"Tug Off\", Default" "Select Your Behavior" {
                            tunnel: w395 -> [_ w403 w409 w412 w418 w423 w429 w435]
                            tunnel: [w398 w404 w410 w414 w417 w424 w430 w436] -> w394
                            tunnel: w393 -> [w398 w402 w406 w415 w419 w425 w431 w437]
                            frame "Tug Off", Default {
                            }
                            frame "Manual Mode" {
                              n103 = To Word Integer(number=w403) -> (16bit integer=w399:cluster{"X":i16, "Y":i16})
                              n104 = call <vilib>:"Draw Line.vi"("picture"=w402, "end point"=w399, "color(black)"=u32 16746732, "pen"=T7 {"Width"=1, "Style"=enum."Solid"}) -> ("new picture"=w404:picture)  [unwired: 5 in]
                            }
                            frame "Back Up" {
                              n105 = To Word Integer(number=w409) -> (16bit integer=w405:cluster{"X":i16, "Y":i16})
                              n106 = call <vilib>:"Draw Line.vi"("picture"=w406, "end point"=w405, "color(black)"=u32 16719872, "pen"=T7 {"Width"=1, "Style"=enum."Dash"}) -> ("new picture"=w410:picture)  [unwired: 5 in]
                            }
                            frame "Left Wall Follow" {
                              n107 = To Word Integer(number=w412) -> (16bit integer=w413:cluster{"X":i16, "Y":i16})
                              n108 = call <vilib>:"Draw Line.vi"("picture"=w415, "end point"=w413, "color(black)"=u32 16769042, "pen"=T7 {"Width"=1, "Style"=enum."Dash"}) -> ("new picture"=w414:picture)  [unwired: 5 in]
                            }
                            frame "Goto WayPoint" {
                              n109 = To Word Integer(number=w418) -> (16bit integer=w420:cluster{"X":i16, "Y":i16})
                              n110 = call <vilib>:"Draw Line.vi"("picture"=w419, "end point"=w420, "color(black)"=u32 60927, "pen"=T7 {"Width"=1, "Style"=enum."Solid"}) -> ("new picture"=w417:picture)  [unwired: 5 in]
                            }
                            frame "Circle" {
                              n111 = To Word Integer(number=w423) -> (16bit integer=w428:cluster{"X":i16, "Y":i16})
                              n112 = call <vilib>:"Draw Line.vi"("picture"=w425, "end point"=w428, "color(black)"=u32 65351, "pen"=T7 {"Width"=1, "Style"=enum."DashDot"}) -> ("new picture"=w424:picture)  [unwired: 5 in]
                            }
                            frame "Right Wall Follow" {
                              n113 = To Word Integer(number=w429) -> (16bit integer=w434:cluster{"X":i16, "Y":i16})
                              n114 = call <vilib>:"Draw Line.vi"("picture"=w431, "end point"=w434, "color(black)"=u32 16754450, "pen"=T7 {"Width"=1, "Style"=enum."Dash"}) -> ("new picture"=w430:picture)  [unwired: 5 in]
                            }
                            frame "Hunt" {
                              n115 = To Word Integer(number=w435) -> (16bit integer=w438:cluster{"X":i16, "Y":i16})
                              n116 = call <vilib>:"Draw Line.vi"("picture"=w437, "end point"=w438, "color(black)"=u32 16720896, "pen"=T7 {"Width"=1, "Style"=enum."DashDotDot"}) -> ("new picture"=w436:picture)  [unwired: 5 in]
                            }
                          }
                        }
                      }
                      n117 = local read "initialized MDF"() -> (w389:T6)
                    }
                    event "Select Your Behavior": Value Change {
                      # "When the user selects a new operation, we disable certain controls that aren't relevant to\nthe operation that the user is performing."
                      n118 = event-data() -> ("NewVal"=w446:T9)  [unwired: 1 in]
                      n119 = property on="Select Pen Attributes" class="Clust (strict)"() -> ("Controls[]"=w445:refnum<vi>[])  [unwired: 2 in, 2 out]
                      n120 = case shown="\"Manual Mode\"" w446 {
                        tunnel: w445 -> [w450 w451 w455 w459 w463 w467 w471 w475]
                        tunnel: "Select Pen Attributes" -> [_ _ _ _ _ _ _ _]
                        frame "Manual Mode" {
                          # "All attributes are valid for this\noperation."
                          n121 = Index Array "Index Array"(array=w450, index=1) -> (element=w448:refnum<vi>)
                          n122 = property on="Property Node" class="Ctl"(reference=w448, "Disabled"=u8 0) -> ()  [unwired: 1 in, 2 out]
                        }
                        frame "Back Up" {
                          # "All attributes are valid for this\noperation."
                          n123 = Index Array(array=w451, index=1) -> (element=w453:refnum<vi>)
                          n124 = property class="Ctl"(reference=w453, "Disabled"=u8 0) -> ()  [unwired: 1 in, 2 out]
                        }
                        frame "Tug Off" {
                          # "All attributes are valid for this\noperation."
                          n125 = Index Array "Index Array"(array=w455, index=1) -> (element=w457:refnum<vi>)
                          n126 = property on="Property Node" class="Ctl"(reference=w457, "Disabled"=u8 0) -> ()  [unwired: 1 in, 2 out]
                        }
                        frame "Left Wall Follow" {
                          # "All attributes are valid for this\noperation."
                          n127 = Index Array "Index Array"(array=w459, index=1) -> (element=w461:refnum<vi>)
                          n128 = property on="Property Node" class="Ctl"(reference=w461, "Disabled"=u8 0) -> ()  [unwired: 1 in, 2 out]
                        }
                        frame "Goto WayPoint" {
                          # "All attributes are valid for this\noperation."
                          n129 = Index Array "Index Array"(array=w463, index=1) -> (element=w465:refnum<vi>)
                          n130 = property on="Property Node" class="Ctl"(reference=w465, "Disabled"=u8 0) -> ()  [unwired: 1 in, 2 out]
                        }
                        frame "Circle" {
                          # "All attributes are valid for this\noperation."
                          n131 = Index Array "Index Array"(array=w467, index=1) -> (element=w469:refnum<vi>)
                          n132 = property on="Property Node" class="Ctl"(reference=w469, "Disabled"=u8 0) -> ()  [unwired: 1 in, 2 out]
                        }
                        frame "Right Wall Follow" {
                          # "All attributes are valid for this\noperation."
                          n133 = Index Array "Index Array"(array=w471, index=1) -> (element=w473:refnum<vi>)
                          n134 = property on="Property Node" class="Ctl"(reference=w473, "Disabled"=u8 0) -> ()  [unwired: 1 in, 2 out]
                        }
                        frame "Hunt" {
                          # "All attributes are valid for this\noperation."
                          n135 = Index Array "Index Array"(array=w475, index=1) -> (element=w477:refnum<vi>)
                          n136 = property on="Property Node" class="Ctl"(reference=w477, "Disabled"=u8 0) -> ()  [unwired: 1 in, 2 out]
                        }
                      }
                      n137 = local read "initialized MDF"() -> (w443:T6)
                    }
                    event "MissionDefFile": Mouse Up {
                      # "When the user is finished drawing, we complete the operation."
                      # "Finished Drawing"
                      n138 = event-data() -> ()  [unwired: 1 in, 3 out]
                      n139 = local write "Draw??"(FALSE ("Draw??")) -> ()
                      n140 = local read "initialized MDF"() -> (w480:T6)
                    }
                  }
                  "MissionDefFile" <- w353
                  "MDF_Original" <- w351
                  n141 = call "UpdateMDF.vi"("Index"=0, "MDF_In"=w351) -> ("MDF_Out"=→"MDF":T6)  [unwired: 9 in]
                }
                n142 = Wait (ms)(milliseconds to wait=u32 200) -> ()  [unwired: 1 out]
                "Way Point Index" <- 0 ("Boundary Point Index")
              }
              frame #1 {
                w484 = T10."AutoMode" ("Tab")
                # "Force \nnext \ncase\nto  be\nAutoMode"
                n143 = local write "Tab"(w484) -> ()
                n144 = local write "Exit Planning"(FALSE ("Exit Planning")) -> ()
              }
            }
          }
          frame "ManualMode" {
            # "Removing map shift register\nfixed memory leak?"
            # "Manual Steering by dashboard heading steering wheel\nand by speed slider"
            # "This mode lets \noperator directly\ndrive robot via\nthe ManualMode\ntabbed interface"
            n145 = while {
              shift-right: [w515] -> _
              shift-left: _ -> [w514]
              tunnel: w489 -> [w507]
              shift-right: [w504] -> _
              shift-left: _ -> [w503]
              tunnel: w487 -> [w501]
              stop <- w513 stop-if-true
              # "WhereAmI?"
              n146 = Get Date/Time In Seconds "GetMiissionCurrentTime"() -> (seconds since 1Jan1904=w508:timestamp)
              n147 = call "WhereForebrainPerception.vi"("Where? Midbrain"="WhereAmI?FromBase") -> ("Where? Forebrain"=→"Where? Manual":T8, "(xr,yr)"=w504:cluster{"X":dbl, "Y":dbl}, "Direction"=w493:dbl)  [unwired: 3 in, 1 out]
              "(xr,yr)" <- w504
              n148 = local read "ManualModeStop"() -> (w513:bool)
              n149 = To Double Precision Float(number=w508) -> (double precision float=w509:dbl)
              n150 = Greater Or Equal?(x=w493, y=181.0) -> (x >= y?=w498:bool)
              n151 = local read "Manual Heading"() -> (w505:i16)
              n152 = Subtract(x=w509, y=w507) -> (x-y=w510:dbl)
              n153 = Not(x=w514) -> (.not. x?=w515:bool)
              n154 = call "DrawRobot.vi"("(xr,yr) old"=w503, "(xr,yr) new"=w504, "2D Picture"=w501) -> ("new picture"=→"ManualMissionMap":picture)
              n155 = Divide(x=w510, y=60.0) -> (x/y=w512:dbl)
              "MissionTime" <- w512
              n156 = Subtract(x=w493, y=360.0) -> (x-y=w496:dbl)
              n157 = shared-variable "My Computer\\RobotBrainExLibrary.lvlib\\MissionTime"(w512) -> ()  [unwired: 1 in, 1 out]
              n158 = Select(t=w496, s=w498, f=w493) -> (s? t:f=w495:dbl)
              n159 = Bundle("Direction"=w495, "Manual Heading"=w505) -> (→"Heading":cluster{"Direction":dbl, "Manual Heading":i16})  [unwired: 1 in]
              n160 = Wait Until Next ms Multiple(millisecond multiple=u32 100 ("milliseconds to wait")) -> ()  [unwired: 1 out]
              "Where? 2" <- w514
            }
            n161 = while {
              shift-right: [w522] -> _
              shift-left: _ -> [w523]
              stop <- "ManualModeStop" stop-if-true
              # "WhatIsAroundMe?"
              n162 = local read "WhatAroundMeMap?"() -> (w517:cluster{"T":dbl, "Range":dbl, "Bearing":dbl}[])
              n163 = call "ProcessLidarData.vi"("WhatAroundMe?MM"=w517) -> ("Collision"=w518:bool, "data array [mag, phase (deg)]"=w519:cluster{"magnitude":dbl, "phase":dbl}[])
              "CollisionLight" <- w518
              n164 = Not(x=w523) -> (.not. x?=w522:bool)
              "MWhat?" <- w522
              n165 = call "SimLIDARPlot.vi"("data array [mag, phase (deg)]"=w519) -> ("SONAR"=→"ManualModeMapDAR":picture)  [unwired: 1 in]
              n166 = case shown="True" w518 {
                frame False {
                  # "No \nBeep"
                }
                frame True {
                  n167 = call <vilib>:"Beep.vi"("use system alert? (T)"=TRUE, "duration (msec)"=u32 1000, "frequency (Hz)"=u32 900) -> ()  [unwired: 9 in]
                }
              }
              n168 = Wait Until Next ms Multiple(millisecond multiple=u32 100 ("milliseconds to wait")) -> ()  [unwired: 1 out]
            }
            n169 = while {
              shift-right: [w547] -> _
              shift-left: _ -> [w546]
              stop <- w545 stop-if-true
              # "HowAmI?"
              n170 = local read "Battery\nVolts"() -> (w544:i16)
              n171 = local read "ManualModeStop"() -> (w545:bool)
              n172 = Not(x=w546) -> (.not. x?=w547:bool)
              n173 = Divide(x=w544, y=i16 1000) -> (x/y=→"Battery":dbl)
              n174 = Wait Until Next ms Multiple(millisecond multiple=u32 100 ("milliseconds to wait")) -> ()  [unwired: 1 out]
              "How? 2" <- w546
            }
            n175 = while {
              shift-right: [w541] -> _
              shift-left: _ -> [w540]
              stop <- w539 stop-if-true
              # "ForebrainAct"
              n176 = local read "E-Stop"() -> (w537:bool)
              n177 = local read "ManualModeStop"() -> (w539:bool)
              n178 = Select(t=0.0, s=w537, f="Manual Vel") -> (s? t:f=w534:dbl)
              n179 = To Word Integer(number=w534) -> (16bit integer=w532:i16)
              "Speed" <- w532
              n180 = local read "Send String"() -> (→"Send String to NXT":string)
              n181 = To Word Integer(number="Behavior Command") -> (16bit integer=w529:i16)
              n182 = local write "Upper Midbrain Active"("Upper Midbrain Active") -> ()
              n183 = local write "Mode"(w529) -> ()
              n184 = local write "Desired \nVelocity"(w532) -> ()
              n185 = local write "Local\nHeading"("Manual Heading") -> ()
              n186 = Not(x=w540) -> (.not. x?=w541:bool)
              n187 = Wait Until Next ms Multiple(millisecond multiple=u32 50 ("milliseconds to wait")) -> ()  [unwired: 1 out]
              "ActManual" <- w540
            }
            n188 = local read "ManualModeStop"() -> (w490:bool)
            n189 = case shown="True" w490 {
              tunnel: [TRUE ("s") w551] -> w492
              tunnel: [T10."ManualMode" ("Tab") w552] -> w491
              frame False {
              }
              frame True {
                # "Debounce tab for clean transition"
                n190 = flat-sequence {
                  tunnel: [w558] -> w552
                  tunnel: [TRUE ("s")] -> w551
                  frame #0 {
                    n191 = Wait (ms)(milliseconds to wait=u32 100) -> ()  [unwired: 1 out]
                  }
                  frame #1 {
                    w558 = T10."Startup&Shutdown" ("Tab")
                    # "Turn off\nVelocity\non \nExit"
                    n192 = local write "ManualModeStop"(FALSE ("ManualModeStop")) -> ()
                    n193 = local write "Desired \nVelocity"(i16 0 ("Desired \nVelocity")) -> ()
                    n194 = local write "Local\nHeading"(i16 0 ("Local\nHeading")) -> ()
                    n195 = local write "Mode"(i16 0 ("Mode")) -> ()
                    n196 = local write "Tab"(w558) -> ()
                  }
                }
              }
            }
          }
          frame "AutoMode" {
            n197 = flat-sequence {
              tunnel: w567 -> [_]
              tunnel: [w570] -> w565
              tunnel: w564 -> [w570]
              tunnel: w563 -> [w569]
              tunnel: [w569] -> w562
              tunnel: w561 -> [_]
              tunnel: w565 -> [w577]
              tunnel: w562 -> [w575]
              tunnel: [w654] -> w568
              tunnel: [FALSE ("s")] -> w566
              frame #0 {
                # "Run Robot\nbased on\nmission\ndefinition\nfile"
                n198 = local write "AutoMissionMap"(w569) -> ()
                n199 = while {
                  shift-right: [w573] -> _
                  shift-left: _ -> [w572]
                  stop <- "RunAutoMode" continue-if-true
                  # "Wait for Run\nbutton press\nbefore\nturning on\nAutoMode\nCode"
                  n200 = Not(x=w572) -> (.not. x?=w573:bool)
                  n201 = Wait Until Next ms Multiple(millisecond multiple=u32 100 ("milliseconds to wait")) -> ()  [unwired: 1 out]
                  "Ready" <- w572
                }
              }
              frame #1 {
                n202 = while {
                  shift-right: [w623] -> _
                  shift-left: _ -> [w614]
                  tunnel: w577 -> [w618]
                  shift-right: [w616] -> _
                  shift-left: _ -> [w617]
                  tunnel: w575 -> [w609]
                  stop <- w613 stop-if-true
                  # "WhereAmI?"
                  n203 = local read "WhereAmI?FromBase"() -> (w608:T8)
                  n204 = Get Date/Time In Seconds "GetMiissionCurrentTime"() -> (seconds since 1Jan1904=w619:timestamp)
                  n205 = call "WhereForebrainPerception.vi"("Where? Midbrain"=w608) -> ("(xr,yr)"=w616:cluster{"X":dbl, "Y":dbl}, "Direction"=w602:dbl)  [unwired: 3 in, 2 out]
                  "Robot Position" <- w616
                  n206 = local read "RunAutoMode"() -> (w613:bool)
                  n207 = Greater Or Equal?(x=w602, y=181.0) -> (x >= y?=w606:bool)
                  n208 = To Double Precision Float(number=w619) -> (double precision float=w620:dbl)
                  n209 = Subtract(x=w620, y=w618) -> (x-y=w621:dbl)
                  n210 = Not(x=w614) -> (.not. x?=w623:bool)
                  n211 = call "DrawRobot.vi"("(xr,yr) old"=w617, "(xr,yr) new"=w616, "2D Picture"=w609) -> ("new picture"=→"AutoMissionMap":picture)
                  n212 = local read "SteerAngle"() -> (w611:dbl)
                  n213 = Divide(x=w621, y=60.0) -> (x/y=w615:dbl)
                  "MissionTimeAuto" <- w615
                  n214 = Subtract(x=w602, y=360.0) -> (x-y=w604:dbl)
                  n215 = Select(t=w604, s=w606, f=w602) -> (s? t:f=w603:dbl)
                  n216 = shared-variable "My Computer\\RobotBrainExLibrary.lvlib\\MissionTime"(w615) -> ()  [unwired: 1 in, 1 out]
                  n217 = Bundle("Direction"=w603, "SteerAngle"=w611) -> (→"A Heading":cluster{"Direction":dbl, "SteerAngle":dbl})  [unwired: 1 in]
                  n218 = Wait Until Next ms Multiple(millisecond multiple=u32 50 ("milliseconds to wait")) -> ()  [unwired: 1 out]
                  "Where?" <- w614
                }
                n219 = while {
                  shift-right: [w644] -> _
                  shift-left: _ -> [w643]
                  shift-right: [w626] -> _
                  shift-left: 0.0 ("SteerAngle") -> [w639]
                  stop <- w646 stop-if-true
                  # "needs to put out heading in local coordinates"
                  # "Think"
                  n220 = Not(x=w643) -> (.not. x?=w644:bool)
                  n221 = Or(x="Pause", y="E-Stop") -> (x .or. y?=w630:bool)
                  n222 = local read "WhereAmI?FromBase"() -> (w642:T8)
                  n223 = local read "WhatAroundMeMap?"() -> (w641:cluster{"T":dbl, "Range":dbl, "Bearing":dbl}[])
                  n224 = local read "MDF"() -> (w632:T6)
                  n225 = call "GotoWaypoint.vi"("InhibitIn"=w630, "CurrentSteerAngle"=w639, "WhatAroundMe? Clean"=w641, "WhereAmI? Clean"=w642, "MDF In"=w632) -> ("BehCom"=→"Current Behavior":T9, "MDF Out"=w634:T6, "ActCommand"=→"WayPointAct":dbl[], "Vel"=w627:dbl, "SteerAngle"=w626:dbl)  [unwired: 1 in, 1 out]
                  "SteerAngle" <- w626
                  "A Speed" <- w627
                  n226 = To Long Integer(number=w627) -> (32bit integer=w628:i32)
                  n227 = To Long Integer(number=w626) -> (32bit integer=w625:i32)
                  n228 = local write "MDF"(w634) -> ()
                  n229 = local write "Desired \nVelocity"(w628) -> ()
                  n230 = local read "RunAutoMode"() -> (w646:bool)
                  n231 = local write "Local\nHeading"(w625) -> ()
                  n232 = local read "MDF_Original"() -> (w637:T6)
                  n233 = local read "MDF"() -> (w636:T6)
                  n234 = Select(t=w637, s="Rerun MDF", f=w636) -> (s? t:f=w633:T6)
                  n235 = local write "MDF"(w633) -> ()
                  n236 = Wait Until Next ms Multiple(millisecond multiple=u32 50 ("milliseconds to wait")) -> ()  [unwired: 1 out]
                  "Neo-C" <- w643
                }
                n237 = while {
                  shift-right: [w595] -> _
                  shift-left: _ -> [w597]
                  stop <- w594 stop-if-true
                  # "WhatIsAroundMe?"
                  n238 = local read "WhatAroundMeMap?"() -> (w591:cluster{"T":dbl, "Range":dbl, "Bearing":dbl}[])
                  n239 = call "ProcessLidarData.vi"("WhatAroundMe?MM"=w591) -> ("Collision"=w592:bool, "data array [mag, phase (deg)]"=w596:cluster{"magnitude":dbl, "phase":dbl}[])
                  "CollisionLight 2" <- w592
                  n240 = local read "RunAutoMode"() -> (w594:bool)
                  n241 = call "SimLIDARPlot.vi"("data array [mag, phase (deg)]"=w596) -> ("SONAR"=→"AutoModeLIDAR":picture)  [unwired: 1 in]
                  n242 = Not(x=w597) -> (.not. x?=w595:bool)
                  "What?" <- w595
                  n243 = case shown="True" w592 {
                    frame False {
                      # "No \nBeep"
                    }
                    frame True {
                      n244 = call <vilib>:"Beep.vi"("use system alert? (T)"=TRUE, "duration (msec)"=u32 1000, "frequency (Hz)"=u32 900) -> ()  [unwired: 9 in]
                    }
                  }
                  n245 = Wait Until Next ms Multiple(millisecond multiple=u32 50 ("milliseconds to wait")) -> ()  [unwired: 1 out]
                }
                n246 = while {
                  shift-right: [w589] -> _
                  shift-left: _ -> [w588]
                  stop <- w587 stop-if-true
                  # "HowAmI?"
                  n247 = local read "Battery\nVolts"() -> (w585:i16)
                  n248 = local read "RunAutoMode"() -> (w587:bool)
                  n249 = Not(x=w588) -> (.not. x?=w589:bool)
                  n250 = Divide(x=w585, y=i16 1000) -> (x/y=→"AutoBattery":dbl)
                  n251 = Wait Until Next ms Multiple(millisecond multiple=u32 80 ("milliseconds to wait")) -> ()  [unwired: 1 out]
                  "How?" <- w588
                }
                n252 = while {
                  shift-right: [w582] -> _
                  shift-left: _ -> [w581]
                  stop <- w580 stop-if-true
                  # "calculate desired heading.vi"
                  # "see calc desired\nheading"
                  # "convert to \noutputtin\nDesired v and\nlocal heading"
                  # "chnage arbiter to be -180 to 180"
                  # "Note:\nadd other beh to\narbiter"
                  # "ForebrainAct"
                  n253 = local read "WayPointAct"() -> (w579:dbl[])
                  n254 = local read "RunAutoMode"() -> (w580:bool)
                  n255 = Not(x=w581) -> (.not. x?=w582:bool)
                  n256 = call "ForebrainArbiter.vi"("WaypointInput"=w579) -> ("ForebrainActCom"=w578:dbl[])  [unwired: 14 in]
                  n257 = shared-variable "My Computer\\RobotBrainExLibrary.lvlib\\ActCommand"(w578) -> ()  [unwired: 1 in, 1 out]
                  n258 = Wait Until Next ms Multiple(millisecond multiple=u32 50 ("milliseconds to wait")) -> ()  [unwired: 1 out]
                  "Act" <- w581
                }
              }
              frame #2 {
                w654 = T10."Startup&Shutdown" ("Tab")
                # "Set robot Vel to 0"
                # "Reset latched run\nswitch"
                # "Force control to\nShutdown Case"
                n259 = shared-variable "My Computer\\RobotBrainExLibrary.lvlib\\ForebrainCom"(T11 {"VelCom"=0.0, "BehCom"=enum."OpenFieldTransit"} ("ForebrainCom")) -> ()  [unwired: 1 in, 1 out]
                n260 = local write "RunAutoMode"(TRUE ("RunAutoMode")) -> ()
                n261 = Initialize Array(0.0 ("element"), 90 ("dimension size")) -> (w650:dbl[])
                n262 = shared-variable "My Computer\\RobotBrainExLibrary.lvlib\\ActCommand"(w650) -> ()  [unwired: 1 in, 1 out]
                n263 = shared-variable "My Computer\\RobotBrainExLibrary.lvlib\\Xstart"(200.0 ("Xstart")) -> ()  [unwired: 1 in, 1 out]
                n264 = shared-variable "My Computer\\RobotBrainExLibrary.lvlib\\Ystart"(400.0 ("Ystart")) -> ()  [unwired: 1 in, 1 out]
                n265 = local write "Tab"(w654) -> ()
              }
            }
          }
          frame "Documentation" {
            # "Add:\n1) Blinking lights in each loop to show that they are running"
            # "This mode is just a static data flow picture of the ForeBrain"
            n266 = Wait (ms)(milliseconds to wait=u32 500) -> ()  [unwired: 1 out]
          }
          frame "DebugTHINK" {
            w666 = T10."Startup&Shutdown" ("Tab")
            # "Add:\n1) a button for each midbrain behavior to help in debugging\n2) graph of \"neural\" arbiter brain waves for each actuator\n3) a button for each forebrain behavior"
            # "Put code here in place of delay"
            # "Sends Tab Control\nback to Startup\ncase"
            n267 = Wait (ms)(milliseconds to wait=u32 5000) -> ()  [unwired: 1 out]
            n268 = local write "Tab"(w666) -> ()
          }
          frame "Basic AutoMode" {
            # "last heading"
            # "if we are under a cloud"
            # "Where am I?\nDraw robots current\n location on map"
            n269 = case shown="2" "MISSION NUMBER (1 OR 2)" {
              tunnel: ["Mission 2" "Mission 1"] -> w701
              frame 2 {
              }
              frame 1, Default {
              }
            }
            n270 = local read "Tug X"() -> (w727:i32)
            n271 = local read "Tug Y"() -> (w728:i32)
            n272 = local read "Current Waypoint"() -> (w702:dbl)
            n273 = Bundle("Tug X"=w727, "Tug Y"=w728) -> (w691:cluster{"Tug X":i32, "Tug Y":i32})  [unwired: 1 in]
            n274 = local read "Buoy Array"() -> (w697:i32[][])
            n275 = case shown="1" "WAYPOINT MODE" {
              tunnel: [w737 w748] -> w715
              tunnel: [w738 w746] -> w714
              tunnel: w701 -> [w736 w742]
              tunnel: w702 -> [w739 w741]
              tunnel: [w733 w740] -> w687
              frame 1 {
                n276 = Array Size(array=w736) -> (size(s)=w735:i32[])
                n277 = call "MidpointGenerator.vi"("Waypoint"=w739, "Array"=w736) -> ("Y"=w737:dbl, "X"=w738:dbl)
                n278 = Index Array(array=w735, index=0) -> (element=w733:i32)
              }
              frame 0, Default {
                # "Index of Destination Point"
                n279 = Array Size(array=w742) -> (size(s)=w744:i32[])
                n280 = Index Array(array=w742, index (row)=w741, index (col)=1 ("disabled index (col)")) -> (element=w747:i64)
                n281 = Index Array(array=w742, index (row)=w741, index (col)=0 ("index (row)")) -> (element=w749:i64)
                n282 = Index Array(array=w744, index=0) -> (element=w740:i32)
                n283 = To Double Precision Float(number=w747) -> (double precision float=w748:dbl)
                n284 = To Double Precision Float(number=w749) -> (double precision float=w746:dbl)
              }
            }
            "Number Waypoints" <- w687
            n285 = call "DrawRobot.vi"("(xr,yr) old"=w691, "(xr,yr) new"=w691, "2D Picture"=w726) -> ("new picture"=w692:picture)
            n286 = local read "Direction"() -> (w693:dbl)
            n287 = call "BuoyRectifier.vi"("Buoy Array"=w697) -> ("Normalized Buoy Array"=w696:i32[][])
            "Normalized Buoy Array" <- w696
            n288 = call "DrawHeading.vi"("(xr,yr) old"=w691, "Heading"=w693, "2D Picture"=w692) -> ("new picture"=w690:picture)
            n289 = call "DrawWaypoints.vi"("Array"=w701, "2D Picture"=w690) -> ("new picture"=w700:picture)  [unwired: 1 in]
            n290 = local read "Buoy Array"() -> (w699:i32[][])
            n291 = local write "Buoy Array"(w696) -> ()
            n292 = call "DrawBuoy.vi"("Array"=w699, "2D Picture"=w700) -> ("new picture"=→"BAM Mission Map":picture)  [unwired: 1 in]
            n293 = local read "WhereAmI?FromBase"() -> (w730:T8)
            n294 = call "unpackGates.vi"("Current Waypoint"=w702, "Destinations Array"=w701) -> ("Past Gate"=w703:i64[], "Current Gate"=w704:i64[])
            n295 = Unbundle(w730) -> ("X"=w677:dbl, "Y"=w676:dbl, "Direction"=w729:dbl)  [unwired: 1 out]
            "Pixel X" <- w677
            "Pixel Y" <- w676
            "Direction" <- w729
            n296 = Less Or Equal To 0?(x=w676) -> (x <= 0?=w684:bool)
            n297 = Not(x=w684) -> (.not. x?=w683:bool)
            n298 = call "crossedLineWayPoint.vi"("X Boat (Pixel)"=w677, "Y Boat (Pixel)"=w676, "Current Gate"=w704, "Past Gate"=w703) -> ()  [unwired: 1 in, 1 out]
            n299 = call "NearWaypointTest.vi"("Yrobot"=w676, "Xrobot"=w677, "Ywaypoint"=w715, "Xwaypoiny"=w714) -> ("AtWaypoint"=w668:bool)  [unwired: 7 in]
            n300 = call "rudderAngle.vi"("BoatHeading"=w729, "YGoal"=w714, "XGoal"=w715, "Yboat"=w677, "Xboat"=w676) -> ("RudderAngle"=w681:i16)  [unwired: 1 in, 2 out]
            n301 = local read "Number Waypoints"() -> (w710:i32)
            n302 = local read "Current Waypoint"() -> (w711:dbl)
            n303 = Select(t="Heading", s="Manual\nOverride", f=w681) -> (s? t:f=w682:i16)
            n304 = local read "Battery\nVolts"() -> (w724:i16)
            n305 = local read "under cloud?"() -> (w689:bool)
            n306 = Select(t=w682, s=w683, f=w685) -> (s? t:f=w678:i16)
            n307 = Select(t=w685, s=w689, f=w681) -> (s? t:f=w694:i16)
            n308 = Increment(x=w711) -> (x+1=w712:dbl)
            n309 = Greater Or Equal?(x=w711, y=w710) -> (x >= y?=w708:bool)
            n310 = Select(t=i16 7, s=w708, f=i16 8 ("t")) -> (s? t:f=w716:i16)
            n311 = call "RandomishWalk.vi"("Y"=w676, "X"=w677, "Alt Rudder"="Alt Rudder", "Default Rudder"="Default Rudder", "Max Radius"="Max Radius") -> ("Rudder Command"=w679:dbl)  [unwired: 1 out]
            n312 = Divide(x=w724, y=1000) -> (x/y=→"Battery Level":dbl)
            n313 = Select(t=w712, s=w668, f=w711) -> (s? t:f=w713:dbl)
            n314 = Select(t=w679, s="Battshit", f=w678) -> (s? t:f=w680:dbl)
            n315 = local write "Current Waypoint"(w713) -> ()
            n316 = Select(t="Velocity", s="Manual\nOverride", f=w716) -> (s? t:f=w671:i16)
            n317 = Bundle("RudderAngle"=w678, "t"=w671, "under cloud?"=w689, "RudderAngle"=w694) -> (→"Forebrain to Midbrain":T16)  [unwired: 1 in]
            n318 = Select(t="Batshit Velocity", s="Battshit", f=w671) -> (s? t:f=w672:i16)
            n319 = local write "Desired \nVelocity"(w672) -> ()
            n320 = local write "Local\nHeading"(w680) -> ()
            n321 = local read "Tab"() -> (w720:T3)
          }
        }
        n322 = Not(x=w228) -> (.not. x?=w212:bool)
        "Robot Live" <- w212
      }
      n323 = while {
        tunnel: w61 -> [w173]
        tunnel: w58 -> [w172]
        tunnel: [w169] -> w59
        tunnel: [w168] -> w60
        stop <- w167 continue-if-true
        # "will lock up main  process\nwaiting for return string"
        # "communication loop with NXT"
        # "send a string to the NXT and receive a String in return"
        n324 = local read "Send String"() -> (w165:string)
        "NXT String Sent" <- w165
        n325 = Wait Until Next ms Multiple(millisecond multiple=u32 200) -> ()  [unwired: 1 out]
        n326 = call "XB PC Send.vi"("error in (no error)"=w172, "String"=w165, "VISA resource name"=w173) -> ("error out"=w171:errorcluster, "return count"=→"return count":u32, "VISA resource name out"=w170:refnum<visa-resource-name>)
        n327 = call "XB PC Hear.vi"("VISA resource name"=w170, "error in (no error)"=w171) -> ("VISA resource name out"=w168:refnum<visa-resource-name>, "String Received"=w164:string, "error out"=w169:errorcluster)
        "NXT String Received" <- w164
        n328 = local read "RunRobot"() -> (w167:bool)
        n329 = local write "String Received"(w164) -> ()
      }
      n330 = while {
        tunnel: w57 -> [w193]
        tunnel: w56 -> [w192]
        tunnel: [w191] -> w54
        tunnel: [w190] -> w55
        shift-right: [w184] -> _
        shift-left: _ -> [w183]
        shift-right: [w182] -> _
        shift-left: _ -> [w181]
        shift-left: _ -> [w180]
        shift-left: _ -> [w179]
        shift-left: _ -> [w176]
        shift-left: _ -> [w175]
        shift-left: _ -> [w174]
        stop <- w194 continue-if-true
        w196 = 250  # timeout
        # "Finds and displays tugs position"
        # "runs continuously till program stops"
        # "Comminications with Base Station"
        # "receive string"
        # "If time out, post timeout and\nremove the timeout error"
        # "Read data from the port."
        n331 = Compound Arithmetic op=OR(w174, w181, w180, w179, w175, w176) -> (w178:bool)
        n332 = Wait Until Next ms Multiple(millisecond multiple=u32 1) -> ()  [unwired: 1 out]
        n333 = Not(x=w178) -> (.not. x?=→"under cloud?":bool)
        n334 = UDP Read(connection ID=w193, timeout ms (25000)=w196, 8:w192) -> (data out=w185:string, error out=w197:errorcluster, 3:w190:refnum<k16>)  [unwired: 1 in, 2 out]
        "Base Station String" <- w185
        n335 = local write "Base Station data rec'd"(w185) -> ()
        n336 = Unbundle By Name(w197) -> ("code"=w200:i32)
        n337 = Equal?(x=w200, y=56) -> (x = y?=w198:bool)
        "BS Time Out?" <- w198
        n338 = case shown="True" w198 {
          tunnel: [w207 errorcluster {"status"=FALSE, "code"=0, "source"=""} ("error out")] -> w191
          tunnel: w197 -> [w207 _]
          frame False {
          }
          frame True {
          }
        }
        n339 = call "PC parse the data.vi"("Nav String"=w185, "Tug"="Tug letter") -> ("Buoy locations"=w189:cluster{"regular expression":string, i32, i32}[], "Tug Location"=w187:T17, "Valid?"=w188:bool)  [unwired: 1 out]
        "Valid ?" <- w188
        n340 = local write "Buoy locations"(w189) -> ()
        n341 = case shown="True" w188 {
          tunnel: w187 -> [_ w206]
          frame False {
            # "No \nchange"
          }
          frame True {
            # "New values from BaseStation"
            n342 = shared-variable "My Computer\\RobotBrainExLibrary.lvlib\\MissionTime"() -> (w205:dbl)  [unwired: 1 in, 1 out]
            n343 = Unbundle(w206) -> (w204:i32, w203:i32, w202:i32)  [unwired: 1 out]
            n344 = local write "Tug X"(w204) -> ()
            n345 = local write "Tug Y"(w203) -> ()
            n346 = local write "Tug H"(w202) -> ()
            n347 = Bundle(w205, w204, w203, w202) -> (w201:cluster{dbl, i32, i32, i32})  [unwired: 1 in]
            n348 = local write "WhereAmI?FromBase"(w201) -> ()
          }
        }
        n349 = local read "RunRobot"() -> (w194:bool)
        n350 = Not(x=w183) -> (.not. x?=w184:bool)
        n351 = local read "Valid ?"() -> (w182:bool)
        "udp rate" <- w183
      }
      n352 = while {
        tunnel: w58 -> [_]
        stop <- w119 continue-if-true
        n353 = local read "Manual\nOverride"() -> (w118:bool)
        n354 = local read "Upper Midbrain Active"() -> (w116:bool)
        n355 = Not(x=w118) -> (.not. x?=w117:bool)
        n356 = And(x=w116, y=w117) -> (x .and. y?=w115:bool)
        n357 = case shown="True" w115 {
          frame False {
            # "loop timimng \ncontrolled externally"
            # "Send commands to NXT"
            n358 = local read "Desired \nVelocity"() -> (w130:i16)
            n359 = local read "Local\nHeading"() -> (w129:i16)
            n360 = local read "Mode"() -> (w128:i16)
            n361 = case shown="2" w128 {
              tunnel: w130 -> [w133 w144 w151]
              tunnel: w129 -> [w132 w143 w152]
              tunnel: [w134 w139 w147] -> w122
              tunnel: i16 7 ("element") -> [w131 w140 w148]
              frame 0, Default {
                w135 = i16 0 ("element")
                n362 = Build Array(u8 91 ("element"), w131, w132, w133, i16 1 ("element"), w135, w135, w135, w135, w135, u8 93 ("element")) -> (w134:i16[])
              }
              frame 1 {
                w141 = i16 0 ("element")
                n363 = Build Array(u8 91 ("element"), w140, w143, w144, w141, i16 1 ("element"), w141, w141, w141, w141, u8 93 ("element")) -> (w139:i16[])
              }
              frame 2 {
                w149 = i16 0 ("element")
                n364 = Build Array(u8 91 ("element"), w148, w152, w151, w149, w149, i16 1 ("element"), w149, w149, w149, u8 93 ("element")) -> (w147:i16[])
              }
            }
            n365 = Select(t=u8[] [91, 7, 7, 7, 1, 0, 0, 0, 0, 0, 92], s="Soft E-Stop", f=w122) -> (s? t:f=w123:i16[])
            n366 = Add(x=w123, y=u8[] [0, 65, 65, 65, 65, 65, 65, 65, 65, 65, 0]) -> (x+y=w124:i16[])
            n367 = Byte Array To String(unsigned byte array=w124) -> (string=w121:string)
            n368 = local write "Send String"(w121) -> ()
          }
          frame True {
            n369 = local read "WhatAroundMeMap? Filtered"() -> (w158:cluster{"T":dbl, "Range":dbl, "Bearing":dbl}[])
            n370 = local read "Ir distance"() -> (w159:i16)
            n371 = local read "Forebrain to Midbrain"() -> (w156:T1)
            n372 = local read "Direction"() -> (w155:dbl)
            n373 = call "UpperMidbrain.vi"("Boat Heading"=w155, "tweak"="Upper Midbrain Tweaks", "WhatAroundMeMap?"=w158, "SOFT E-STOP"="SOFT E-STOP", "behavior weights"="Midbrain Behavior weights", "ir distance"=w159, "ForeBrain to Midbrain"=w156) -> ("string"=w157:string)  [unwired: 4 in]
            n374 = local write "Send String"(w157) -> ()
          }
        }
        n375 = local read "RunRobot"() -> (w119:bool)
      }
      n376 = while {
        tunnel: w58 -> [_]
        stop <- w86 continue-if-true
        # "Receive information from NXT"
        n377 = local read "String Received"() -> (w91:string)
        n378 = Wait Until Next ms Multiple(millisecond multiple=u32 100) -> ()  [unwired: 1 out]
        n379 = String Subset(string=w91, offset (0)=1, length (rest)=1 ("length (rest)")) -> (substring=w90:string)
        n380 = case shown="Default" w90 {
          tunnel: w91 -> [w92 w100]
          frame Default {
            n381 = Search/Split String(string=w92, search string/char (-)=",", offset (0)=1) -> (substring before match=w94:string)  [unwired: 2 out]
            n382 = Decimal String To Number(string=w94, offset=1) -> (number=w96:i32)  [unwired: 1 in, 1 out]
            n383 = To Word Integer(number=w96) -> (16bit integer=→"Ir distance":i16)
          }
          frame "N" {
            # "0-15"
            # "Parse command \"N\""
            n384 = String Subset(string=w100, offset (0)=2, length (rest)=4 ("length (rest)")) -> (substring=w111:string)
            n385 = String Subset(string=w100, offset (0)=6, length (rest)=3 ("length (rest)")) -> (substring=w107:string)
            n386 = String Subset(string=w100, offset (0)=9, length (rest)=2 ("length (rest)")) -> (substring=w103:string)
            n387 = Decimal String To Number(string=w111) -> (number=w114:i32)  [unwired: 2 in, 1 out]
            n388 = Decimal String To Number(string=w107) -> (number=w106:i32)  [unwired: 2 in, 1 out]
            n389 = Decimal String To Number(string=w103) -> (number=w104:i32)  [unwired: 2 in, 1 out]
            n390 = To Word Integer(number=w114) -> (16bit integer=w110:i16)
            n391 = To Word Integer(number=w106) -> (16bit integer=w105:i16)
            n392 = To Long Integer(number=w104) -> (32bit integer=w99:i32)
            n393 = local write "LidarDist"(w105) -> ()
            n394 = local write "Battery\nVolts"(w110) -> ()
            n395 = local write "IR Index"(w99) -> ()
          }
        }
        n396 = local read "RunRobot"() -> (w86:bool)
      }
      n397 = while {
        shift-right: [w71] -> _
        shift-left: _ -> [w78]
        shift-left: _ -> [w79]
        shift-left: _ -> [w80]
        stop <- w85 continue-if-true
        # "Run Simulated MapDAR"
        n398 = local read "Tug X"() -> (w83:i32)
        n399 = local read "Tug Y"() -> (w82:i32)
        n400 = local read "Tug H"() -> (w81:i32)
        n401 = local read "Buoy Array"() -> (w76:i32[][])
        n402 = call "FilterLidar.vi"("WhatAroundMeMap? Last 2"=w80, "WhatAroundMeMap? Last 3"=w79, "WhatAroundMeMap? Last"=w78) -> ("WhatAroundMeMap?"=→"WhatAroundMeMap? Filtered":cluster{"T":dbl, "Range":dbl, "Bearing":dbl}[])  [unwired: 8 in]
        n403 = Bundle "Bundle"("Tug X"=w83, "Tug Y"=w82, "Tug H"=w81) -> (w84:cluster{"Tug X":i32, "Tug Y":i32, "Tug H":i32})  [unwired: 1 in]
        n404 = call "HindbrainLIDAR_Sim.vi"("Buoys"=w76, "SubPosition"=w84) -> ("WhatAroundMe"=w73:cluster{"T":dbl, "Range":dbl, "Bearing":dbl}[], "WhatAroundMe?Walls"=w72:cluster{"T":dbl, "Range":dbl, "Bearing":dbl}[])
        n405 = Not(x="MapDarWithBuoys?") -> (.not. x?=w74:bool)
        n406 = local read "RunRobot"() -> (w85:bool)
        n407 = Select(t=w72, s=w74, f=w73) -> (s? t:f=w71:cluster{"T":dbl, "Range":dbl, "Bearing":dbl}[])
        "WhatAroundMeMap?" <- w71
      }
    }
    frame #2 {
      # "Close XBee Radio"
      # "Close UDP port"
      # "Realease LIDAR\nMemory"
      # "Reset Run \nSwitch"
      # "Shutdown Robot"
      n408 = call "Pixel_LIDAR_Close.vi"("error in (no error) 2"=w755, "Image"=w756) -> ()  [unwired: 1 in]
      n409 = local write "RunRobot"(TRUE ("RunRobot")) -> ()
      n410 = call "XB PC Close.vi"("error in (no error)"=w753, "VISA resource name"=w754) -> ()
      n411 = UDP Close(connection ID=w752, 8:w751) -> ()  [unwired: 2 out]
      "error out" <- w753
    }
  }
